vi "MoD Main-Optimize - HPLC - SUZUKI 04122017.vi"() -> ()   [LabVIEW 2015]
uses:
  <vilib>/ni845x/ni845x.llb/ni845xControl.ctl
  <vilib>/MakerHub/LINX/Public/Peripherals/Analog/Analog Read 1 Chan.vi
  <vilib>/MakerHub/LINX/Public/Peripherals/Analog/Analog Read N Chans.vi
  <vilib>/MakerHub/LINX/Public/Peripherals/Digital/Digital Write 1 Chan.vi
  <vilib>/MakerHub/LINX/Private/Local IO/LinxAnalogRead.vi
  <vilib>/MakerHub/LINX/Public/Utilities/Check Channel.vi
  <vilib>/MakerHub/LINX/Public/Peripherals/Digital/Digital Write N Chans.vi
  <vilib>/MakerHub/LINX/Private/Local IO/LinxDigitalWrite.vi
  <vilib>/addons/control/pid/pid.llb/PID Control Input Filter (DBL).vi
  <vilib>/MakerHub/LINX/Private/Utilties/Generate Error.vi
  <vilib>/addons/control/pid/autopid.llb/PID Online Autotuning (Relay Feedback).vi
  <vilib>/ni845x/ni845x.llb/NI-845x Close Device Reference.vi
  <vilib>/MakerHub/LINX/LMH-LINX.lvlib
  <vilib>/addons/control/pid/NI_PID_autopid.lvlib
  <vilib>/addons/control/pid/NI_PID_pid.lvlib
  <instrlib>/Harvard Apparatus PHD Ultra Series/Harvard Apparatus PHD Ultra Series.lvlib
panel:
  in  "Debug_run_button":bool
  out "Phase_Sensor_voltage":dbl
  out "P_tot":dbl
  out "pause for ms":bool=TRUE
  out "stop_xl_write":bool=TRUE
  out "Num_exp_till_pause":i32
  out "Syringe_pump?":bool=TRUE
  out "System Error":bool=TRUE
  out "error out":errorcluster
  out "Pump setpoint(ul/min) 6":dbl format="%#_13g"
  out "Pump setpoint(ul/min) 5":dbl format="%#_13g"
  out "Pump setpoint(ul/min) 4":dbl format="%#_13g"
  out "Pump setpoint(ul/min) 3":dbl format="%#_13g"
  out "Pump setpoint(ul/min) 2":dbl format="%#_13g"
  out "Pump setpoint(ul/min) 1":dbl format="%#_13g"
  out "Volume (ul) 5":dbl format="%#_13g"
  out "Volume (ul) 4":dbl format="%#_13g"
  out "Volume (ul) 3":dbl format="%#_13g"
  out "Volume (ul) 2":dbl format="%#_13g"
  out "Volume (ul) 1":dbl format="%#_13g"
  in  "tau 5":dbl format="%#_13g"
  out "tau 4":dbl format="%#_13g"
  out "tau 3":dbl format="%#_13g"
  out "tau 2":dbl format="%#_13g"
  out "tau 1":dbl format="%#_13g"
  out "Reactor Length":dbl format="%#_13g"
  out "Flowrate Sensor 2":dbl format="%#_13g"
  out "Flowrate Sensor 1":dbl format="%#_13g"
  out "Pressure 2":dbl format="%#_13g"
  out "Pressure 1":dbl format="%#_13g"
  out "Temperature Control 5":bool=TRUE
  out "Temperature Control 4":bool=TRUE
  out "Temperature Control 3":bool=TRUE
  out "Temperature Control 2":bool=TRUE
  out "Temperature Control 1":bool=TRUE
  out "Temperature SP 5":dbl format="%#_g'C"
  out "Temperature SP 4":dbl format="%#_g'C"
  out "Temperature SP 3":dbl format="%#_g'C"
  out "Temperature SP 2":dbl format="%#_g'C"
  out "Temperature SP 1":dbl format="%#_g'C"
  in  "Bay Temperature 5":dbl
  in  "SSR Duration 5":dbl
  in  "SSR Duration 4":dbl
  in  "SSR Duration 3":dbl
  in  "SSR Duration 2":dbl
  in  "SSR Duration 1":dbl
  in  "Total Product Amount":dbl=1.0 format="%#_gml"
  out "Setup Error":bool=TRUE
  out "Error Message":string
  out "ID CTR":i32
  in  "Tab Control 2":enum32{"Faults", "Devices"}(tab)=enum."Devices"
  out "Fault Cluster":T1
  in  "COMM Port:: Harvard Syringe Pump":refnum<visa-resource-name>="COM5"
  in  "Sample Valve COMM::Port":refnum<visa-resource-name>="COM6"
  in  "Arduino COMM Port":refnum<visa-resource-name>="COM3"
  in  "COMM Port :: Milligat Pumps":refnum<visa-resource-name>="COM10"
  in  "IR Sensor Device":T2="USB0::0x3923::0x7514::01B3FF21::RAW"
  in  "Tab Control":enum32{"Setup", "Parameters", "Monitoring"}(tab)
  in  "System decide help Button":bool
  in  "Reaction Scheme Confirm":bool
  in  "Synthesis Route Array":string[](array[string])=["3-Br-Pyridine _ Biphenyl", "K2CO3", "PhB(OH)2", "", "", ""]
  in  "Manual/Automated":bool
  in  "Save Button":bool
  in  "Open Button":bool
  in  "New rxn scheme button":bool
  in  "System decide help Button 2":bool
  out "Setup Confirm":bool=TRUE
  in  "BAY 1":u16(ring) items=["                 Bypass", "             Hot Reactor", "               Separator"]
  in  "BAY 5":u16(ring) items=["                     Bypass", "                Hot Reactor", "                 Separator"]
  in  "BAY 4":u16(ring) items=["                     Bypass", "                Hot Reactor", "                  Separator"]
  in  "BAY 3":u16(ring)=1 items=["                     Bypass", "                 Hot Reactor", "                  Separator"]
  in  "BAY 2":u16(ring) items=["                     Bypass", "                Hot Reactor", "                  Separator"]
  in  "System Parameters Help Button":bool
  in  "System Parameters Confirm Button":bool
  in  "Bay Parameters":T3={"Pump 1 Reagent Concentration"=0.8, "Pump 2 Reagent Concentration"=0.55, "Pump 3 Reagent Concentration"=0.4, "Pump 4 Reagent Concentration"=0.0, "Pump 5 Reagent Concentration"=0.0, "Bay 1 Parameters"={"Pump 1 Flowrate"=0.0, "optimize_temp"=FALSE, "optimize_tau"=TRUE, "Run at set flowrate"=FALSE, "Pump 2 Flowrate"=0.0, "Temperature Params"=[0.0, 40.0, 100.0], "pump params 1"=[0.0, 32.5, 325.0], "pump params 2"=[0.0, 32.5, 325.0]}, "Bay 2 Parameters"={"Pump 3 Flowrate"=0.0, "optimize_temp"=FALSE, "optimize_tau"=TRUE, "Run at set flowrate"=FALSE, "Temperature Params"=[0.0, 40.0, 100.0], "Resisdence time params"=[0.0, 65.0, 650.0], "pump_at_ratio"=FALSE, "pump_num_ratio"=0.0}, "Bay 3 Parameters"={"Pump 4 Flowrate"=0.0, "optimize_temp"=TRUE, "optimize_tau"=FALSE, "Run at set flowrate"=FALSE, "Temperature Params"=[0.0, 40.0, 100.0], "Resisdence time params"=[0.0, 0.0, 0.0], "pump_at_ratio"=FALSE, "pump_num_ratio"=0.0}, "Bay 4 Parameters"={"Pump 5 Flowrate"=40.0, "Run at set flowrate"=FALSE, "optimize_temp"=FALSE, "optimize_tau"=FALSE, "Resisdence time params"=[0.0, 36.0, 225.0], "Temperature Params"=[0.0, 40.0, 80.0], "pump_at_ratio"=FALSE, "pump_num_ratio"=0.0}, "Bay 5 Parameters"={"Pump 6 Flowrate"=0.0, "Run at set flowrate"=FALSE, "optimize_temp"=FALSE, "optimize_tau"=FALSE, "Resisdence time params"=[0.0, 0.0, 0.0], "Temperature Params"=[0.0, 0.0, 0.0], "pump_at_ratio"=FALSE, "pump_num_ratio"=0.2}, "Bay 1 Flow Rate Ratio \n(Pump 1: Pump 2)"=1.0, "tube_id(in)"=[enum.".02", enum.".03", enum.".03", enum.".03", enum.".03"], "xml_filename"="temp_xml", "Excel File Name"="C:\\Users\\HPLC\\Dropbox (MIT)\\MoD Files\\Data\\HWE Results\\SUZUKI Optimization HPLC - 04122017", "hplc File Name"="C:\\Chem32\\1\\Data\\MOD", "Matlab File"="C:\\Users\\HPLC\\Dropbox (MIT)\\MoD Files\\Data\\SUZUKI 04132017b", "Syringe for Pump 2?"=FALSE, "Num_conditons_per_wait"=1.0, "Continue from previous optimization?"=FALSE, "Pump 6 Reagent Concentration"=0.0, "Pause before analysis?"=FALSE, "Hplc Wait time(min)"=9.2} {"Hplc Wait time(min)" format="%#_13g"; "Pump 6 Reagent Concentration" format="%#_6gM"; "Bay 5 Parameters"."Temperature Params" format="%#_g'C"; "Bay 4 Parameters"."Temperature Params" format="%#_g'C"; "Bay 3 Parameters"."Temperature Params" format="%#_g'C"; "Bay 2 Parameters"."Temperature Params" format="%#_g'C"; "Bay 1 Parameters"."Temperature Params" format="%#_g'C"; "Pump 5 Reagent Concentration" format="%#_6gM"; "Pump 4 Reagent Concentration" format="%#_6gM"; "Pump 3 Reagent Concentration" format="%#_6gM"; "Pump 2 Reagent Concentration" format="%#_6gM"; "Pump 1 Reagent Concentration" format="%#_6gM"}
  out "System Confirm Not Clicked":string
  out "Setup Confirm 2":bool=TRUE
  out "Current Experiment":dbl
  in  "Total Number of Experiments":dbl=33.0
  out "Phase Sensor Chart":T4(graph)
  out "HPLC Analysis":bool
  out "Equlibrating Temperature":bool
  out "Flushing System":bool
  out "Calculate condition":bool
  out "System Flush Wait Time":u8(slide) scale=0.0..1149.042355163602
  out "Temperature 5":dbl format="%#_g'C"
  out "Temperature 4":dbl format="%#_g'C"
  out "Temperature 3":dbl format="%#_g'C"
  out "Temperature 2":dbl format="%#_g'C"
  out "Temperature 1":dbl format="%#_g'C"
  out "Flowrate Chart":T4(graph)
  out "Bay 5":u16(ring) items=["                     Bypass", "                   Reactor1", "               Separator"]
  out "Bay 4":u16(ring) items=["                     Bypass", "                   Reactor1", "               Separator"]
  out "Bay 3":u16(ring) items=["                     Bypass", "                   Reactor1", "               Separator"]
  out "Bay 2":u16(ring) items=["                     Bypass", "                   Reactor1", "               Separator"]
  out "Bay 1":u16(ring) items=["                     Bypass", "                   Reactor1", "               Separator"]
  out "Teperature Chart":T4(graph)
  out "Pump Setpoints Chart":T4(graph)
  out "Pressure Chart":T4(graph)
  out "Optimization_loop_index":i32
  out "curr_wait_time":dbl
  out "total_flush_time":dbl
  out "Temp SS? 5":bool=TRUE
  out "Temp SS? 4":bool=TRUE
  out "Temp SS? 3":bool=TRUE
  out "Temp SS? 2":bool=TRUE
  out "Temp SS? 1":bool=TRUE
  out "System Flushed?":bool
  out "stop_button clicked":bool
  out "Total System Resisdence Time(min)":dbl
  out "Stop":bool=TRUE
  in  "Run_Stop_cluster":T5
  # "Molecules on Demand"
  # "Synthesis Route"
  # "Reagent List"
  # "1"
  # "2"
  # "1"
  # "3"
  # "2"
  # "4"
  # "3"
  # "5"
  # "4"
  # "6"
  # "5"
  # "Product"
  # "6"
  # "Have system decide based on synthesis route"
  # "Manually enter bay configuration"
  # "System Schematic"
  # "Optimization Parameters"
  # "Bay"
  # "Tube ID (in)"
  # "1."
  # "2."
  # "3."
  # "4."
  # "5."
  # "Pause after"
  # "Experiments"
  # "Reporting"
  # "XML Output File Name"
  # "Excel Output File Name"
  # "HPLC File Path"
  # "MATLAB File Path"
  # "Temperature"
  # "Flowrate(ul/min)"
  # "Setpoint"
  # "Lower Bound"
  # "Upper Bound"
  # "Optimize?"
  # "-or-"
  # "Run at"
  # "times incoming flow"
  # "Temperature"
  # "Flowrate(ul/min)"
  # "Setpoint"
  # "Lower Bound"
  # "Upper Bound"
  # "Optimize?"
  # "-or-"
  # "Run at"
  # "times incoming flow"
  # "Temperature"
  # "Flowrate(ul/min)"
  # "Setpoint"
  # "Lower Bound"
  # "Upper Bound"
  # "Optimize?"
  # "-or-"
  # "Run at"
  # "times incoming flow"
  # "Temperature"
  # "Flowrate 3 (ul/min)"
  # "Setpoint"
  # "Lower Bound"
  # "Upper Bound"
  # "Optimize?"
  # "-or-"
  # "Run at"
  # "times incoming flow"
  # "Temperature"
  # "Flowrate 1(ul/min)"
  # "Flowrate 2(ul/min)"
  # "Setpoint"
  # "Lower Bound"
  # "Upper Bound"
  # "Optimize?"
  # "Temperature('C)"
  # "Pressure (psi)"
  # "Flowrate (ul/min)"
  # "Pump Flowrate Setpoints(ul/min)"
  # "Phase Sensor Value"
  # "Experimental Steps"
  # "Calculated new conditions"
  # "Flushed System"
  # "Analyzed HPLC"
  # "Equilibrated Temperature"
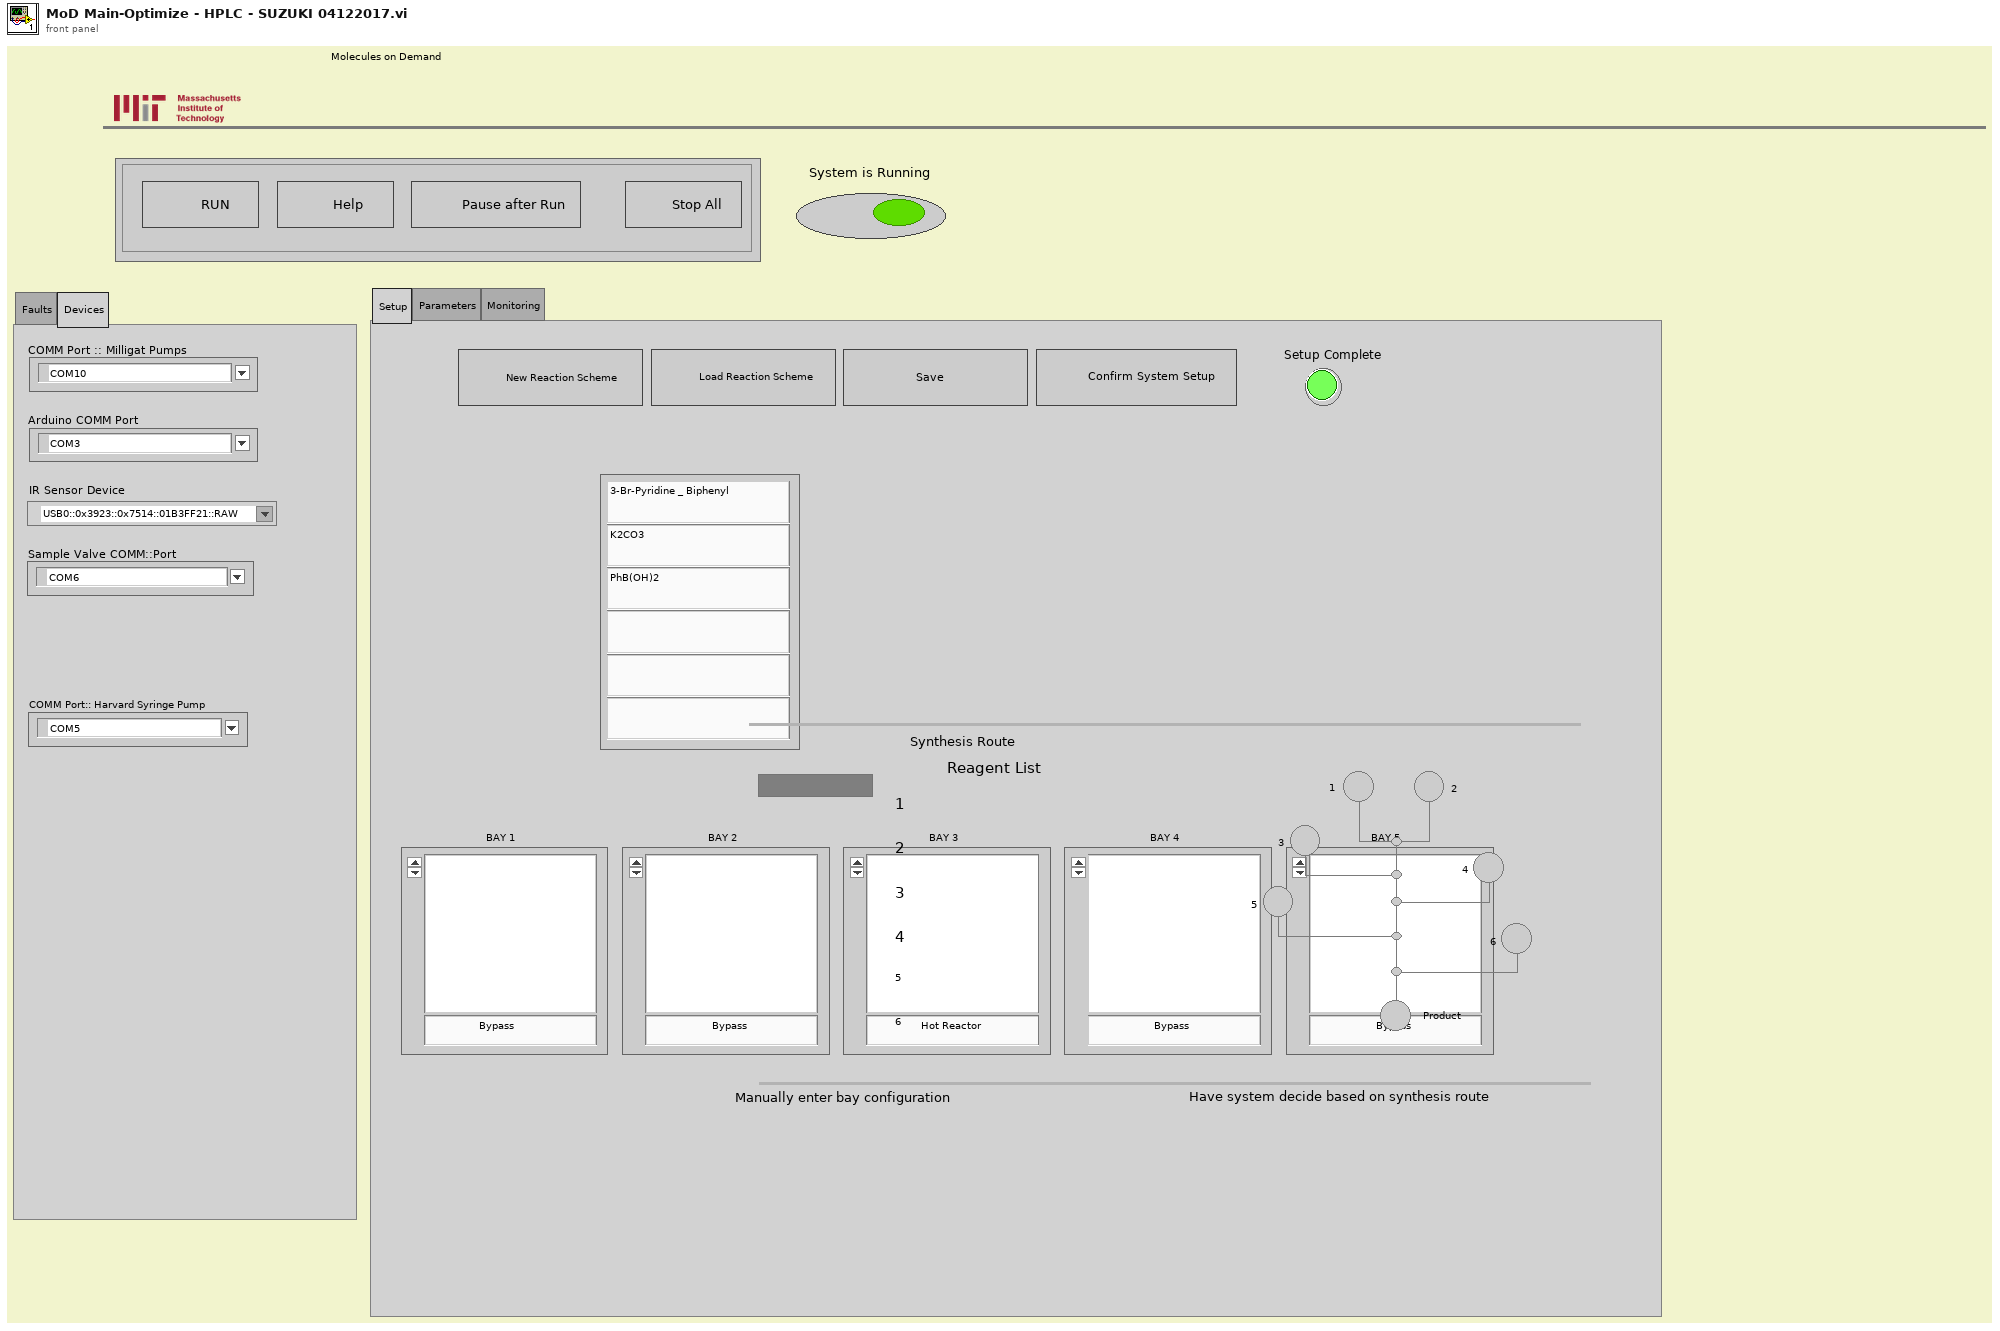
[diagram p1: front panel]
types:
  T1 = cluster{"Pump COMM Port":bool, "Pressure":bool, "Flow Rate":bool, "Temperature Sensor COMM Port":bool, "Arduino COMM Port":bool, "Chiller COMM Port":bool}
  T2 = typedef "ni845xControl.ctl" = refnum<k21>
  T3 = cluster{"Pump 1 Reagent Concentration":dbl, "Pump 2 Reagent Concentration":dbl, "Pump 3 Reagent Concentration":dbl, "Pump 4 Reagent Concentration":dbl, "Pump 5 Reagent Concentration":dbl, "Bay 1 Parameters":cluster{"Pump 1 Flowrate":dbl, "optimize_temp":bool, "optimize_tau":bool, "Run at set flowrate":bool, "Pump 2 Flowrate":dbl, "Temperature Params":dbl[], "pump params 1":dbl[], "pump params 2":dbl[]}, "Bay 2 Parameters":cluster{"Pump 3 Flowrate":dbl, "optimize_temp":bool, "optimize_tau":bool, "Run at set flowrate":bool, "Temperature Params":dbl[], "Resisdence time params":dbl[], "pump_at_ratio":bool, "pump_num_ratio":dbl}, "Bay 3 Parameters":cluster{"Pump 4 Flowrate":dbl, "optimize_temp":bool, "optimize_tau":bool, "Run at set flowrate":bool, "Temperature Params":dbl[], "Resisdence time params":dbl[], "pump_at_ratio":bool, "pump_num_ratio":dbl}, "Bay 4 Parameters":cluster{"Pump 5 Flowrate":dbl, "Run at set flowrate":bool, "optimize_temp":bool, "optimize_tau":bool, "Resisdence time params":dbl[], "Temperature Params":dbl[], "pump_at_ratio":bool, "pump_num_ratio":dbl}, "Bay 5 Parameters":cluster{"Pump 6 Flowrate":dbl, "Run at set flowrate":bool, "optimize_temp":bool, "optimize_tau":bool, "Resisdence time params":dbl[], "Temperature Params":dbl[], "pump_at_ratio":bool, "pump_num_ratio":dbl}, "Bay 1 Flow Rate Ratio \n(Pump 1: Pump 2)":dbl, "tube_id(in)":enum16{".01", ".02", ".03", ".04"}[], "xml_filename":string, "Excel File Name":string, "hplc File Name":string, "Matlab File":string, "Syringe for Pump 2?":bool, "Num_conditons_per_wait":dbl, "Continue from previous optimization?":bool, "Pump 6 Reagent Concentration":dbl, "Pause before analysis?":bool, "Hplc Wait time(min)":dbl}
  T4 = cluster{"[0]":dbl, "[1]":dbl, "[2]":dbl, "[3]":dbl, "[4]":dbl, "[5]":dbl, "[6]":dbl, "[7]":dbl, "[8]":dbl}
  T5 = cluster{"Stop":bool, "Help Button":bool, "Run":bool, "Stop Run Button":bool}
  T6 = cluster{"Proportional gain Kc":dbl, "Integral time Ti (sec)":dbl, "Derivative time Ti (sec)":dbl}
  T7 = cluster{"type of controller":enum16{"P", "PI", "PID"}, "relay cycles":i32, "relay amplitude":dbl, "control specifications":enum16{"Fast", "Normal", "Slow"}, "PV noise level":dbl}
  T8 = typedef "LMH-LINX.lvlib/LINX Ref.ctl" = cluster{"IO":T9, "Interface":T10, "LINX Device Config":T11}
  T9 = typedef "LMH-LINX.lvlib/Platform.ctl" = enum16{"Remote", "Local"}
  T10 = typedef "LMH-LINX.lvlib/Interface.ctl" = enum16{"Serial", "TCP"}
  T11 = typedef "LMH-LINX.lvlib/Device.lvlib/LINX Device Config.ctl" = cluster{"Interface":T10, "COM Port":refnum<visa-resource-name>, "TCP Configuration":T12, "Device Family":u8, "Device ID":u8, "Device Name":string, "TCP Ref":refnum<k5>, "Channels":T13}
  T12 = typedef "LMH-LINX.lvlib/Device.lvlib/TCP Config.ctl" = cluster{"IP Address":string, "Port":u16}
  T13 = typedef "LMH-LINX.lvlib/Channels.ctl" = cluster{"DI":u8[], "DO":u8[], "AI":u8[], "AO":u8[], "PWM":u8[], "QE":u8[], "UART":u8[], "I2C 2":u8[], "SPI":u8[], "CAN":u8[], "Servo":u8[], "AI Ref (V)":dbl, "AI Resolution (Bits)":u8, "AO Ref (V)":dbl, "AO Resolution (Bits)":u8}
  T14 = cluster{"proportional gain (Kc)":dbl, "integral time (Ti, min)":dbl, "derivative time (Td, min)":dbl}
  T15 = enum16{"Left Button", "Center Button", "Right Button", "Window Close"}
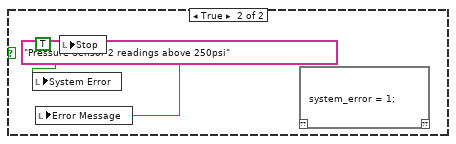
[diagram p2: hidden frame]
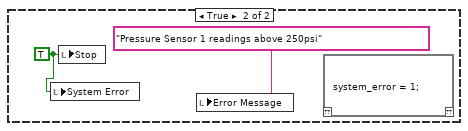
[diagram p3: hidden frame]
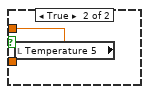
[diagram p4: hidden frame]
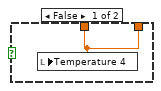
[diagram p5: hidden frame]
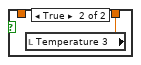
[diagram p6: hidden frame]
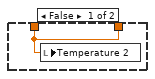
[diagram p7: hidden frame]
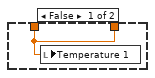
[diagram p8: hidden frame]
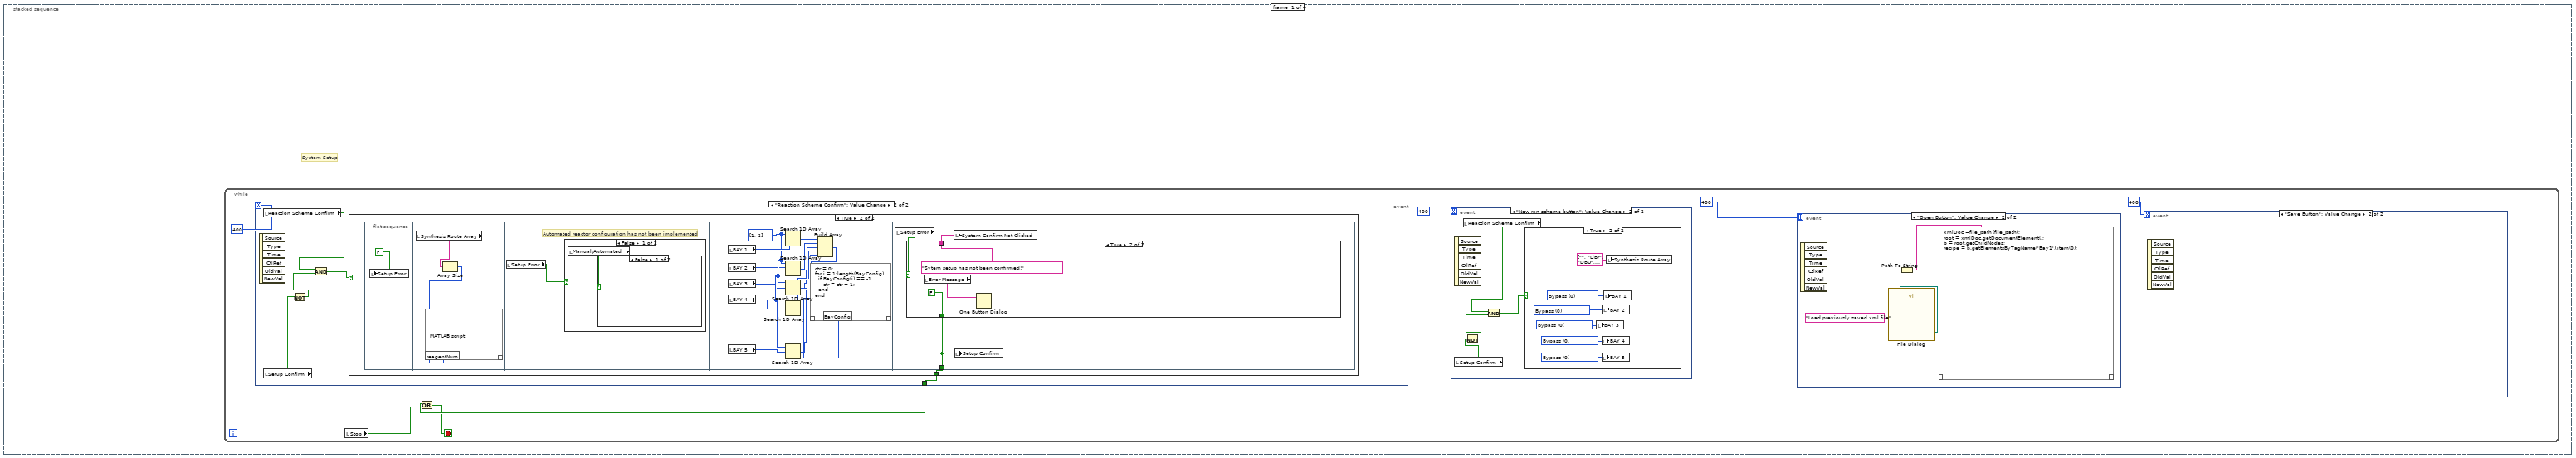
[diagram p9: hidden frame]
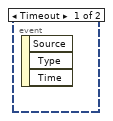
[diagram p10: hidden frame]
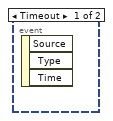
[diagram p11: hidden frame]
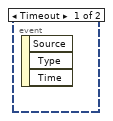
[diagram p12: hidden frame]
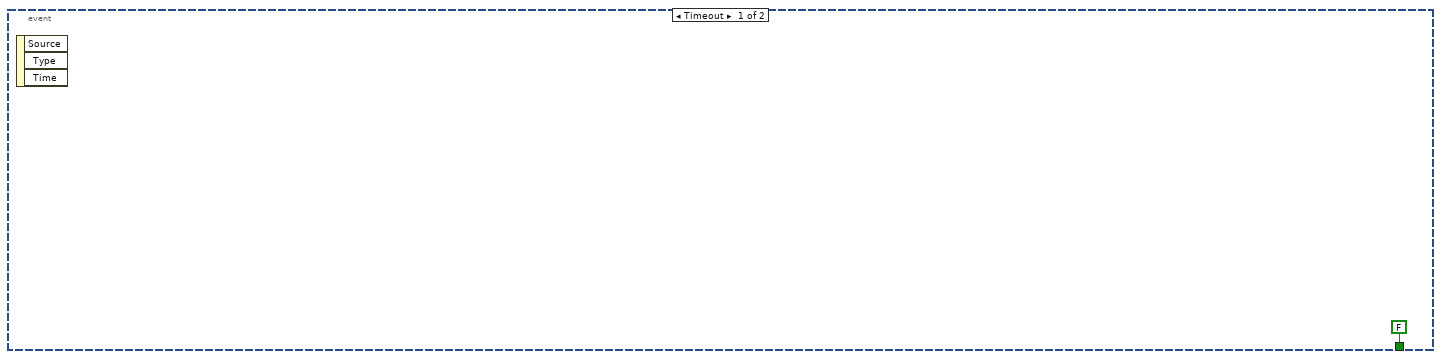
[diagram p14: hidden frame]
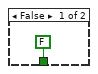
[diagram p15: hidden frame]
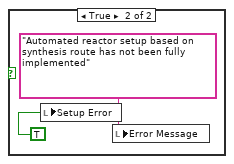
[diagram p16: hidden frame]
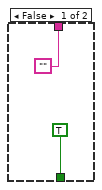
[diagram p18: hidden frame]
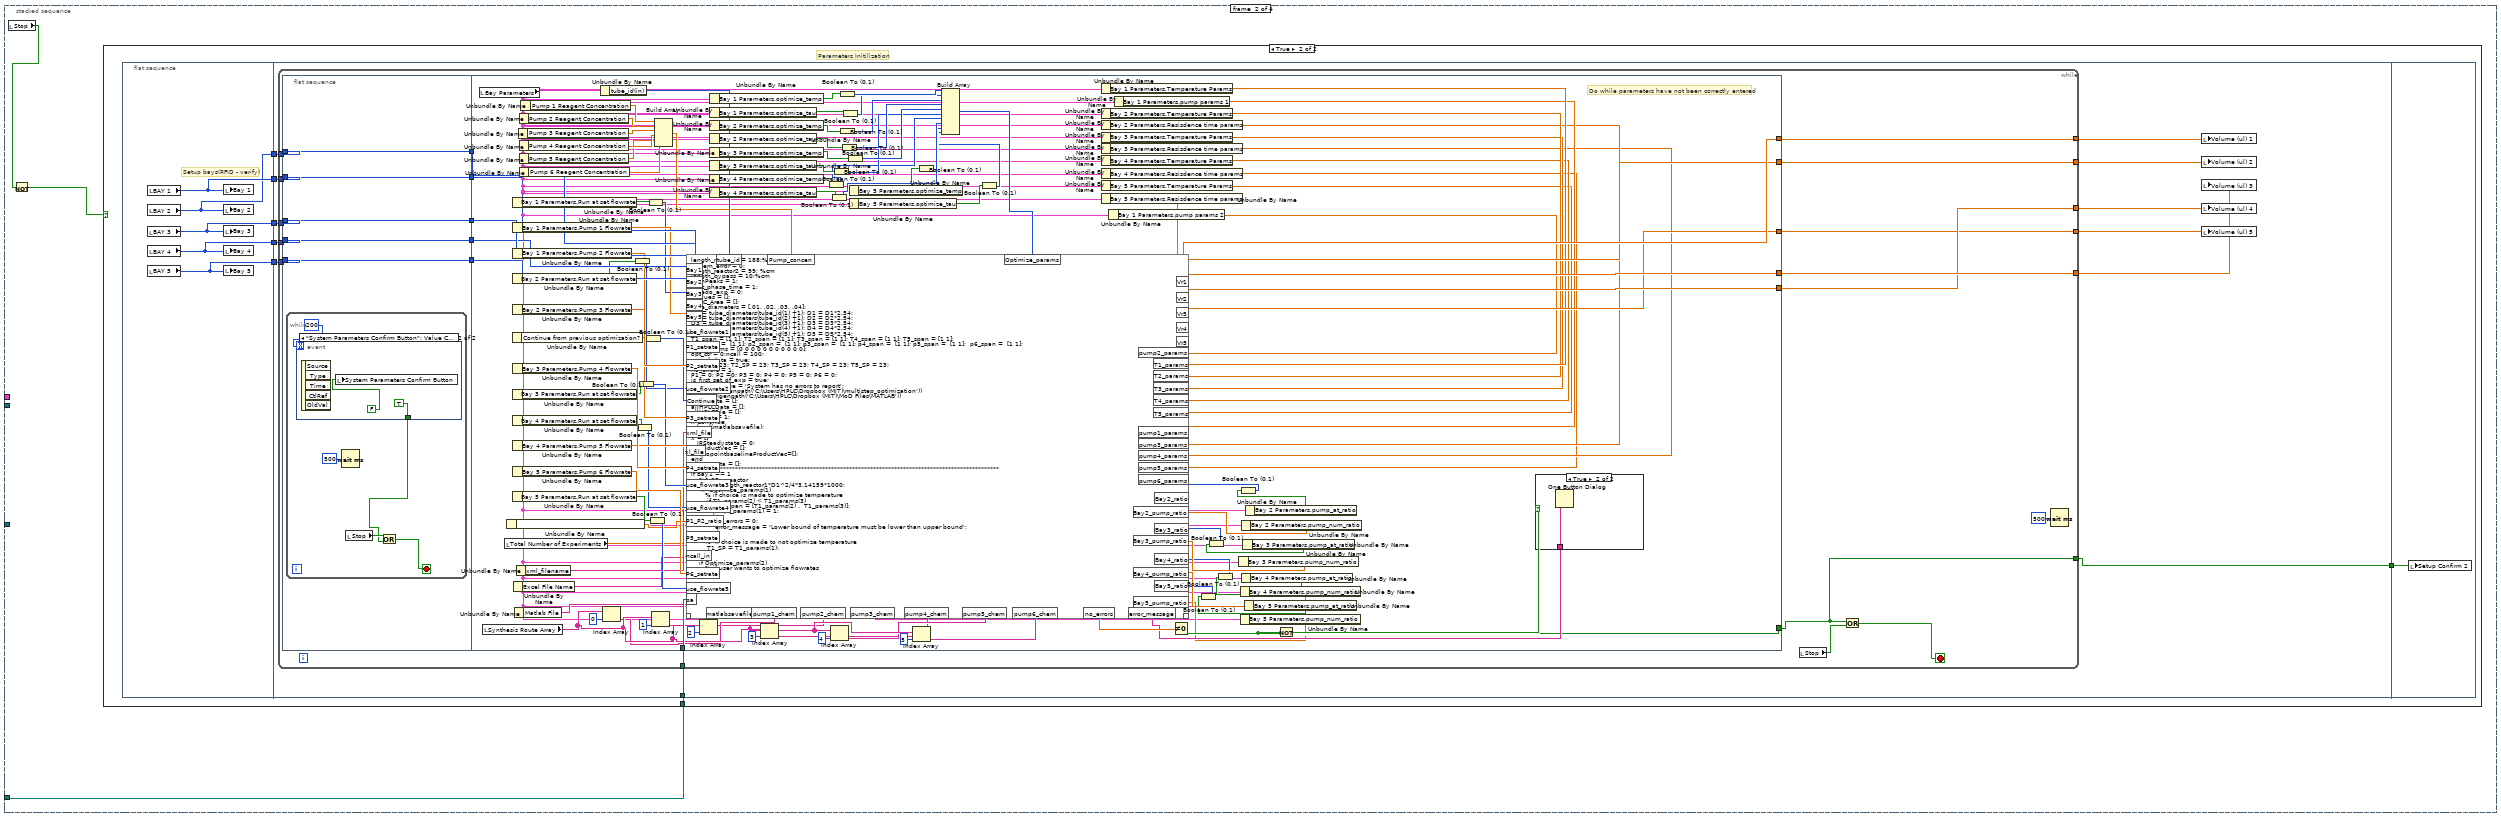
[diagram p19: hidden frame]
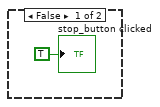
[diagram p20: hidden frame]
diagram:
  # "Assume User always uses the first bay first"
  n1 = flat-sequence {
    tunnel: ["COMM Port :: Milligat Pumps"] -> w10
    tunnel: ["Arduino COMM Port"] -> w9
    tunnel: [w12] -> w2
    tunnel: ["Bay Parameters"] -> w1
    tunnel: [w51] -> w11
    tunnel: w10 -> [w51]
    tunnel: w9 -> [w50]
    tunnel: [w44] -> w8
    tunnel: [w44] -> w7
    tunnel: [w32] -> w4
    tunnel: [w30] -> w3
    tunnel: w2 -> [w30]
    tunnel: w1 -> [w28]
    tunnel: w11 -> [w59]
    tunnel: w8 -> [w58]
    tunnel: w7 -> [w52]
    tunnel: [w57] -> w6
    tunnel: w4 -> [w56]
    tunnel: w3 -> [w53]
    tunnel: w6 -> [w1229]
    tunnel: [w1229] -> w5
    tunnel: w5 -> [w1236]
    frame #0 {
      w16 = FALSE ("Equlibrating Temperature")
      n2 = script code="TempArr1=[23 23 23 23 23 23 23 23 23 23]';\nTempArr2=[23 23 23 23 23 23 23 23 23 23]';\nTempArr3=[23 23 23 23 23 23 23 23 23 23]';\nTempArr4=[23 23 23 23 23 23 23 23 23 23]';\nTempArr5=[23 23 23 23 23 23 23 23 23 23]';\ntemp_error1 =0;\ntemp_error2 =0;\ntemp_error3 =0;\ntemp_error4 =0;\ntemp_error5 =0;\ntemp_check1 = 0;\ntemp_check2 = 0;\ntemp_check3 = 0;\ntemp_check4 = 0;\ntemp_check5 = 0;\nT1=23;\nT2=23;\nT3=23;\nT4=23;\nT5=23;"() -> ()  [unwired: 1 in, 1 out]
      n3 = call <vilib>:"Initialize.vi"("VISA resource name"="COMM Port:: Harvard Syringe Pump") -> ("VISA resource name out"=w12:refnum<visa-resource-name>)  [unwired: 9 in, 1 out]
      "Stop" <- FALSE ("Stop")
      "ID CTR" <- 0
      "Setup Confirm" <- FALSE ("Setup Confirm")
      "Setup Error" <- FALSE ("Setup Error")
      "Reactor Length" <- 10.5
      "System Error" <- FALSE ("System Error")
      "Num_exp_till_pause" <- 0 ("Num_exp_till_pause")
      "Equlibrating Temperature" <- w16
      "Calculate condition" <- w16
      "Flushing System" <- w16
      "HPLC Analysis" <- w16
      "Setup Confirm 2" <- FALSE ("Setup Confirm 2")
      "stop_xl_write" <- FALSE ("stop_xl_write")
    }
    frame #1 {
      w43 = 23
      (unwired) path "C:/Users/User1/Documents/Lab/MoD/Images"
      n4 = local write "Debug_run_button"(TRUE) -> ()
      n5 = local read "BAY 2"() -> (w48:u16)
      n6 = local read "BAY 3"() -> (w47:u16)
      n7 = local read "BAY 4"() -> (w46:u16)
      n8 = local read "BAY 5"() -> (w45:u16)
      n9 = local read "BAY 1"() -> (w49:u16)
      n10 = local write "Bay 1"(w49) -> ()
      n11 = local write "Bay 2"(w48) -> ()
      n12 = local write "Bay 3"(w47) -> ()
      n13 = local write "Bay 4"(w46) -> ()
      n14 = local write "BAY 5"(w45) -> ()
      n15 = call <vilib>:"Initialize.vi"("Serial Port"=w50) -> ("LINX Resource"=w44:T8)  [unwired: 8 in, 2 out]
      n16 = Unbundle By Name(w28) -> ("Syringe for Pump 2?"=→"Syringe_pump?":bool)
      n17 = local write "Temperature 1"(w43) -> ()
      n18 = local write "Temperature 2"(w43) -> ()
      n19 = local write "Temperature 3"(w43) -> ()
      n20 = local write "Temperature 4"(w43) -> ()
      n21 = local write "Temperature 5"(w43) -> ()
      n22 = local write "Temperature SP 1"(w43) -> ()
      n23 = local write "Temperature SP 2"(w43) -> ()
      n24 = local write "Temperature SP 3"(w43) -> ()
      n25 = local write "Temperature SP 4"(w43) -> ()
      n26 = local write "Temperature SP 5"(w43) -> ()
      n27 = Unbundle By Name(w28) -> ("Pause before analysis?"=→"pause for ms":bool)
      n28 = Current VI's Path() -> (path=w36:path)
      n29 = Strip Path(path=w36) -> (stripped path=w34:path)  [unwired: 1 out]
      n30 = Strip Path(path=w34) -> (stripped path=w33:path)  [unwired: 1 out]
      n31 = Build Path(base path=w33, name or relative path="MATLAB") -> (appended path=w32:path)
      "Pump setpoint(ul/min) 1" <- 0.0 ("Pump setpoint(ul/min) 1")
      "Pump setpoint(ul/min) 2" <- 0.0 ("Pump setpoint(ul/min) 2")
      "Pump setpoint(ul/min) 3" <- 0.0 ("Pump setpoint(ul/min) 3")
      "Pump setpoint(ul/min) 4" <- 0.0 ("Pump setpoint(ul/min) 4")
      "Pump setpoint(ul/min) 5" <- 0.0 ("Pump setpoint(ul/min) 5")
      "Pump setpoint(ul/min) 6" <- 0.0 ("Pump setpoint(ul/min) 6")
    }
    frame #2 {
      # "Main Help Dialog Popup"
      n32 = while {
        stop <- w1224 stop-if-true
        n33 = event shown="[1] \"Run_Stop_cluster.Help Button\": Value Change" {
          selector: _ -> [_ _ _ _ _ _]
          dyn-events: _ -> [_ _ _ _ _ _]
          timeout: 100 -> [_ _ _ _ _ _]
          event Timeout {
            n34 = event-data() -> ()  [unwired: 1 in, 3 out]
          }
          event "Run_Stop_cluster.Help Button": Value Change {
            n35 = local read "Run_Stop_cluster"() -> (w1227:T5)
            n36 = event-data() -> ()  [unwired: 1 in, 4 out]
            n37 = Unbundle By Name(w1227) -> ("Help Button"=w1226:bool)
            n38 = case shown="True" w1226 {
              frame False {
              }
              frame True {
                n39 = call "help.vi"() -> ()  [unwired: 11 in]
              }
            }
          }
          event "System decide help Button": Value Change {
            n40 = event-data() -> ()  [unwired: 1 in, 5 out]
            n41 = call "help_synthesis_man-auto_instructions.vi"() -> ()  [unwired: 12 in]
          }
          event "System Parameters Help Button": Value Change {
            n42 = event-data() -> ()  [unwired: 1 in, 5 out]
            n43 = call "help_parameters_setup.vi"() -> ()  [unwired: 12 in]
          }
          event "System decide help Button 2": Value Change {
            n44 = event-data() -> ()  [unwired: 1 in, 5 out]
            n45 = call "help_synthesis_route_instructions.vi"() -> ()  [unwired: 12 in]
          }
          event "Run_Stop_cluster.Stop": Value Change {
            n46 = event-data() -> ()  [unwired: 1 in, 5 out]
            n47 = local write "Stop"(TRUE) -> ()
          }
        }
        n48 = local read "Stop"() -> (w1224:bool)
      }
      n49 = stacked-sequence {
        tunnel: w59 -> [_ _ _ _]
        tunnel: w58 -> [_ _ _ w424]
        tunnel: [_ _ _ w424] -> w57
        tunnel: w56 -> [_ w258 _ _]
        tunnel: w53 -> [_ _ _ w425]
        frame #0 {
          # "System Setup"
          n50 = while {
            stop <- w204 stop-if-true
            n51 = event shown="[1] \"Reaction Scheme Confirm\": Value Change" {
              selector: _ -> [_ _]
              dyn-events: _ -> [_ _]
              timeout: 400 -> [_ _]
              tunnel: [FALSE w222] -> w206
              event Timeout {
                n52 = event-data() -> ()  [unwired: 1 in, 3 out]
              }
              event "Reaction Scheme Confirm": Value Change {
                n53 = event-data() -> ()  [unwired: 1 in, 6 out]
                n54 = local read "Reaction Scheme Confirm"() -> (w226:bool)
                n55 = local read "Setup Confirm"() -> (w224:bool)
                n56 = Not(x=w224) -> (.not. x?=w223:bool)
                n57 = And(x=w226, y=w223) -> (x .and. y?=w225:bool)
                n58 = case shown="True" w225 {
                  tunnel: [FALSE w228] -> w222
                  frame False {
                  }
                  frame True {
                    n59 = flat-sequence {
                      tunnel: [w248] -> w228
                      frame #0 {
                        n60 = local write "Setup Error"(FALSE) -> ()
                      }
                      frame #1 {
                        n61 = local read "Synthesis Route Array"() -> (w231:string[])
                        n62 = Array Size(array=w231) -> (size(s)=w230:i32)
                        n63 = script code="MATLAB script"("reagentNum"=w230) -> ()  [unwired: 1 in, 1 out]
                      }
                      frame #2 {
                        # "Automated reactor configuration has not been implemented"
                        n64 = local read "Setup Error"() -> (w232:bool)
                        n65 = case shown="False" w232 {
                          frame False {
                            n66 = local read "Manual/Automated"() -> (w233:bool)
                            n67 = case shown="False" w233 {
                              frame False {
                              }
                              frame True {
                                n68 = local write "Setup Error"(TRUE ("Setup Error")) -> ()
                                n69 = local write "Error Message"("Automated reactor setup based on synthesis route has not been fully implemented") -> ()
                              }
                            }
                          }
                          frame True {
                          }
                        }
                      }
                      frame #3 {
                        w246 = i32[] [1, 2]
                        n70 = local read "BAY 1"() -> (w247:u16)
                        n71 = local read "BAY 2"() -> (w245:u16)
                        n72 = local read "BAY 3"() -> (w244:u16)
                        n73 = local read "BAY 4"() -> (w243:u16)
                        n74 = local read "BAY 5"() -> (w242:u16)
                        n75 = Search 1D Array(1D array=w246, element=w247) -> (index of element=w241:i32)  [unwired: 1 in]
                        n76 = Search 1D Array(1D array=w246, element=w245) -> (index of element=w240:i32)  [unwired: 1 in]
                        n77 = Search 1D Array(1D array=w246, element=w244) -> (index of element=w239:i32)  [unwired: 1 in]
                        n78 = Search 1D Array(1D array=w246, element=w243) -> (index of element=w238:i32)  [unwired: 1 in]
                        n79 = Search 1D Array(1D array=w246, element=w242) -> (index of element=w237:i32)  [unwired: 1 in]
                        n80 = Build Array(w241, w240, w239, w238, w237) -> (w236:i32[])
                        n81 = script code="ctr = 0;\nfor i = 1:length(BayConfig)\n  if BayConfig(i) == -1\n     ctr = ctr + 1;\n  end\nend"("BayConfig"=w236) -> ()  [unwired: 1 in, 1 out]
                      }
                      frame #4 {
                        n82 = local read "Setup Error"() -> (w250:bool)
                        n83 = case shown="True" w250 {
                          tunnel: [TRUE FALSE] -> w248
                          tunnel: ["" "Sytem setup has not been confirmed!"] -> w249
                          frame False {
                          }
                          frame True {
                            n84 = local read "Error Message"() -> (w255:string)
                            n85 = One Button Dialog(message=w255) -> ()  [unwired: 1 in, 1 out]
                          }
                        }
                        n86 = local write "System Confirm Not Clicked"(w249) -> ()
                        n87 = local write "Setup Confirm"(w248) -> ()
                      }
                    }
                  }
                }
              }
            }
            n88 = local read "Stop"() -> (w205:bool)
            n89 = Or(x=w206, y=w205) -> (x .or. y?=w204:bool)
            n90 = event shown="[1] \"New rxn scheme button\": Value Change" {
              selector: _ -> [_ _]
              dyn-events: _ -> [_ _]
              timeout: 400 -> [_ _]
              event Timeout {
                n91 = event-data() -> ()  [unwired: 1 in, 3 out]
              }
              event "New rxn scheme button": Value Change {
                n92 = event-data() -> ()  [unwired: 1 in, 6 out]
                n93 = local read "Setup Confirm"() -> (w211:bool)
                n94 = local read "Reaction Scheme Confirm"() -> (w212:bool)
                n95 = Not(x=w211) -> (.not. x?=w214:bool)
                n96 = And(x=w212, y=w214) -> (x .and. y?=w213:bool)
                n97 = case shown="True" w213 {
                  frame False {
                  }
                  frame True {
                    w215 = u16 0 items=["                     Bypass", "                Hot Reactor", "                 Separator"] ("BAY 5")
                    w216 = u16 0 items=["                     Bypass", "                Hot Reactor", "                  Separator"] ("BAY 4")
                    w217 = u16 0 items=["                     Bypass", "                 Hot Reactor", "                  Separator"] ("BAY 3")
                    w218 = u16 0 items=["                     Bypass", "                Hot Reactor", "                  Separator"] ("BAY 2")
                    w219 = u16 0 items=["                 Bypass", "             Hot Reactor", "               Separator"] ("BAY 1")
                    n98 = local write "BAY 3"(w217) -> ()
                    n99 = local write "BAY 4"(w216) -> ()
                    n100 = local write "BAY 5"(w215) -> ()
                    n101 = local write "BAY 2"(w218) -> ()
                    n102 = local write "BAY 1"(w219) -> ()
                    n103 = local write "Synthesis Route Array"(string[] ["", "LiBr", "DBU", "Aldehyde", "Water", "Toluene"] ("Synthesis Route Array")) -> ()
                  }
                }
              }
            }
            n104 = event shown="[1] \"Open Button\": Value Change" {
              selector: _ -> [_ _]
              dyn-events: _ -> [_ _]
              timeout: 400 -> [_ _]
              event Timeout {
                n105 = event-data() -> ()  [unwired: 1 in, 3 out]
              }
              event "Open Button": Value Change {
                n106 = event-data() -> ()  [unwired: 1 in, 6 out]
                n107 = call "File Dialog"("prompt"="Load previously saved xml file") -> ("selected path"=w209:path)  [unwired: 11 in, 3 out]
                n108 = Path To String(path=w209) -> (string=w208:string)
                n109 = script code="xmlDoc = xmlread(file_path);\nroot = xmlDoc.getDocumentElement();\nb = root.getChildNodes;\nrecipe = b.getElementsByTagName('Bay1').item(0);"("file_path"=w208) -> ()  [unwired: 1 in, 1 out]
              }
            }
            n110 = event shown="[1] \"Save Button\": Value Change" {
              selector: _ -> [_ _]
              dyn-events: _ -> [_ _]
              timeout: 400 -> [_ _]
              event Timeout {
                n111 = event-data() -> ()  [unwired: 1 in, 3 out]
              }
              event "Save Button": Value Change {
                n112 = event-data() -> ()  [unwired: 1 in, 6 out]
              }
            }
          }
        }
        frame #1 {
          n113 = local read "Stop"() -> (w257:bool)
          n114 = Not(x=w257) -> (.not. x?=w256:bool)
          n115 = case shown="True" w256 {
            tunnel: w258 -> [_ w261]
            frame False {
              "stop_button clicked" <- TRUE ("stop_button clicked")
            }
            frame True {
              # "Parameters Initilization"
              n116 = flat-sequence {
                tunnel: [w271] -> w266
                tunnel: [w270] -> w265
                tunnel: [w269] -> w264
                tunnel: [w268] -> w263
                tunnel: [w267] -> w262
                tunnel: w266 -> [w283]
                tunnel: w265 -> [w282]
                tunnel: w264 -> [w281]
                tunnel: w263 -> [w280]
                tunnel: w262 -> [w279]
                tunnel: w261 -> [w273]
                tunnel: [w272] -> w260
                tunnel: w260 -> [w422]
                frame #0 {
                  # "Setup bays(RFID - verify)"
                  n117 = local read "BAY 1"() -> (w271:u16)
                  n118 = local read "BAY 2"() -> (w270:u16)
                  n119 = local read "BAY 3"() -> (w269:u16)
                  n120 = local read "BAY 4"() -> (w268:u16)
                  n121 = local read "BAY 5"() -> (w267:u16)
                  n122 = local write "Bay 1"(w271) -> ()
                  n123 = local write "Bay 2"(w270) -> ()
                  n124 = local write "Bay 3"(w269) -> ()
                  n125 = local write "Bay 4"(w268) -> ()
                  n126 = local write "Bay 5"(w267) -> ()
                }
                frame #1 {
                  n127 = while {
                    tunnel: w283 -> [w303]
                    tunnel: w282 -> [w302]
                    tunnel: w281 -> [w301]
                    tunnel: w280 -> [w300]
                    tunnel: w279 -> [w299]
                    tunnel: [w298] -> w278
                    tunnel: [w297] -> w277
                    tunnel: [w296] -> w276
                    tunnel: [w295] -> w275
                    tunnel: [w294] -> w274
                    tunnel: w273 -> [w285]
                    tunnel: [w284] -> w272
                    stop <- w293 stop-if-true
                    n128 = flat-sequence {
                      tunnel: w299 -> [w304]
                      tunnel: w300 -> [w305]
                      tunnel: w301 -> [w306]
                      tunnel: w302 -> [w307]
                      tunnel: w303 -> [w308]
                      tunnel: [w308] -> w290
                      tunnel: [w307] -> w289
                      tunnel: [w306] -> w288
                      tunnel: [w305] -> w287
                      tunnel: [w304] -> w286
                      tunnel: [w408] -> w298
                      tunnel: [w407] -> w297
                      tunnel: [w406] -> w296
                      tunnel: [w405] -> w295
                      tunnel: [w404] -> w294
                      tunnel: [w360] -> w284
                      tunnel: w290 -> [w420]
                      tunnel: w289 -> [w419]
                      tunnel: w288 -> [w418]
                      tunnel: w287 -> [w417]
                      tunnel: w286 -> [w416]
                      tunnel: w285 -> [w356]
                      frame #0 {
                        n129 = while {
                          stop <- w312 stop-if-true
                          n130 = event shown="[1] \"System Parameters Confirm Button\": Value Change" {
                            selector: _ -> [_ _]
                            dyn-events: _ -> [_ _]
                            timeout: u32 200 ("milliseconds to wait") -> [_ _]
                            tunnel: [FALSE TRUE] -> w310
                            event Timeout {
                              n131 = event-data() -> ()  [unwired: 1 in, 3 out]
                            }
                            event "System Parameters Confirm Button": Value Change {
                              n132 = event-data() -> ()  [unwired: 1 in, 5 out]
                              n133 = local write "System Parameters Confirm Button"(FALSE) -> ()
                            }
                          }
                          n134 = Wait (ms)(milliseconds to wait=u32 500) -> ()  [unwired: 1 out]
                          n135 = local read "Stop"() -> (w313:bool)
                          n136 = Or(x=w313, y=w310) -> (x .or. y?=w312:bool)
                        }
                      }
                      frame #1 {
                        # "Do while parameters have not been correctly entered"
                        n137 = local read "Bay Parameters"() -> (w318:T3)
                        n138 = local read "Synthesis Route Array"() -> (w333:string[])
                        n139 = local read "Total Number of Experiments"() -> (w319:dbl)
                        n140 = Unbundle By Name(w318) -> ("Bay 1 Flow Rate Ratio \n(Pump 1: Pump 2)"=w359:dbl)
                        n141 = Unbundle By Name(w318) -> ("Continue from previous optimization?"=w355:bool)
                        n142 = Unbundle By Name(w318) -> ("Bay 1 Parameters.Run at set flowrate"=w403:bool)
                        n143 = Unbundle By Name(w318) -> ("Bay 1 Parameters.Pump 1 Flowrate"=w414:dbl)
                        n144 = Unbundle By Name(w318) -> ("Bay 1 Parameters.Pump 2 Flowrate"=w413:dbl)
                        n145 = Unbundle By Name(w318) -> ("Bay 2 Parameters.Run at set flowrate"=w401:bool)
                        n146 = Unbundle By Name(w318) -> ("Bay 2 Parameters.Pump 3 Flowrate"=w412:dbl)
                        n147 = Unbundle By Name(w318) -> ("Bay 3 Parameters.Pump 4 Flowrate"=w411:dbl)
                        n148 = Unbundle By Name(w318) -> ("Bay 3 Parameters.Run at set flowrate"=w400:bool)
                        n149 = Unbundle By Name(w318) -> ("Bay 4 Parameters.Run at set flowrate"=w397:bool)
                        n150 = Unbundle By Name(w318) -> ("Bay 4 Parameters.Pump 5 Flowrate"=w410:dbl)
                        n151 = Unbundle By Name(w318) -> ("Bay 5 Parameters.Pump 6 Flowrate"=w409:dbl)
                        n152 = Unbundle By Name(w318) -> ("Bay 5 Parameters.Run at set flowrate"=w396:bool)
                        n153 = Unbundle By Name(w318) -> ("Excel File Name"=w357:string)
                        n154 = Unbundle By Name(w318) -> ("Matlab File"=w353:string)
                        n155 = Unbundle By Name(w318) -> ("xml_filename"=w358:string)
                        n156 = Unbundle By Name(w318) -> ("Pump 3 Reagent Concentration"=w324:dbl)
                        n157 = Unbundle By Name(w318) -> ("Pump 2 Reagent Concentration"=w325:dbl)
                        n158 = Unbundle By Name(w318) -> ("Pump 4 Reagent Concentration"=w323:dbl)
                        n159 = Unbundle By Name(w318) -> ("Pump 5 Reagent Concentration"=w322:dbl)
                        n160 = Unbundle By Name(w318) -> ("Pump 6 Reagent Concentration"=w321:dbl)
                        n161 = Unbundle By Name(w318) -> ("Pump 1 Reagent Concentration"=w326:dbl)
                        n162 = Unbundle By Name(w318) -> ("tube_id(in)"=w415:enum16{".01", ".02", ".03", ".04"}[])
                        n163 = Index Array(array=w333, index=0) -> (element=w332:string)
                        n164 = Boolean To (0,1)(Boolean=w401) -> (0, 1=w352:i16)
                        n165 = Boolean To (0,1)(Boolean=w397) -> (0, 1=w398:i16)
                        n166 = Boolean To (0,1)(Boolean=w400) -> (0, 1=w399:i16)
                        n167 = Boolean To (0,1)(Boolean=w355) -> (0, 1=w354:i16)
                        n168 = Boolean To (0,1)(Boolean=w403) -> (0, 1=w402:i16)
                        n169 = Boolean To (0,1)(Boolean=w396) -> (0, 1=w395:i16)
                        n170 = Index Array(array=w333, index=1) -> (element=w327:string)
                        n171 = Build Array(w326, w325, w324, w323, w322, w321) -> (w320:dbl[])
                        n172 = Index Array(array=w333, index=2) -> (element=w328:string)
                        n173 = Unbundle By Name(w318) -> ("Bay 1 Parameters.optimize_temp"=w394:bool)
                        n174 = Unbundle By Name(w318) -> ("Bay 1 Parameters.optimize_tau"=w392:bool)
                        n175 = Unbundle By Name(w318) -> ("Bay 2 Parameters.optimize_temp"=w390:bool)
                        n176 = Unbundle By Name(w318) -> ("Bay 2 Parameters.optimize_tau"=w388:bool)
                        n177 = Unbundle By Name(w318) -> ("Bay 3 Parameters.optimize_temp"=w386:bool)
                        n178 = Unbundle By Name(w318) -> ("Bay 3 Parameters.optimize_tau"=w384:bool)
                        n179 = Unbundle By Name(w318) -> ("Bay 4 Parameters.optimize_temp"=w382:bool)
                        n180 = Unbundle By Name(w318) -> ("Bay 4 Parameters.optimize_tau"=w380:bool)
                        n181 = Index Array(array=w333, index=3) -> (element=w329:string)
                        n182 = Boolean To (0,1)(Boolean=w382) -> (0, 1=w381:i16)
                        n183 = Boolean To (0,1)(Boolean=w380) -> (0, 1=w379:i16)
                        n184 = Index Array(array=w333, index=4) -> (element=w330:string)
                        n185 = Boolean To (0,1)(Boolean=w384) -> (0, 1=w383:i16)
                        n186 = Boolean To (0,1)(Boolean=w390) -> (0, 1=w389:i16)
                        n187 = Boolean To (0,1)(Boolean=w394) -> (0, 1=w393:i16)
                        n188 = Boolean To (0,1)(Boolean=w388) -> (0, 1=w387:i16)
                        n189 = Boolean To (0,1)(Boolean=w392) -> (0, 1=w391:i16)
                        n190 = Boolean To (0,1)(Boolean=w386) -> (0, 1=w385:i16)
                        n191 = Unbundle By Name(w318) -> ("Bay 5 Parameters.optimize_temp"=w378:bool)
                        n192 = Unbundle By Name(w318) -> ("Bay 5 Parameters.optimize_tau"=w376:bool)
                        n193 = Index Array(array=w333, index=5) -> (element=w331:string)
                        n194 = Boolean To (0,1)(Boolean=w378) -> (0, 1=w377:i16)
                        n195 = Boolean To (0,1)(Boolean=w376) -> (0, 1=w375:i16)
                        n196 = Build Array(w393, w391, w389, w387, w385, w383, w381, w379, w377, w375) -> (w374:i16[])
                        n197 = Unbundle By Name(w318) -> ("Bay 1 Parameters.Temperature Params"=w371:dbl[])
                        n198 = Unbundle By Name(w318) -> ("Bay 2 Parameters.Temperature Params"=w370:dbl[])
                        n199 = Unbundle By Name(w318) -> ("Bay 2 Parameters.Resisdence time params"=w365:dbl[])
                        n200 = Unbundle By Name(w318) -> ("Bay 3 Parameters.Temperature Params"=w369:dbl[])
                        n201 = Unbundle By Name(w318) -> ("Bay 3 Parameters.Resisdence time params"=w364:dbl[])
                        n202 = Unbundle By Name(w318) -> ("Bay 4 Parameters.Temperature Params"=w368:dbl[])
                        n203 = Unbundle By Name(w318) -> ("Bay 4 Parameters.Resisdence time params"=w363:dbl[])
                        n204 = Unbundle By Name(w318) -> ("Bay 5 Parameters.Temperature Params"=w367:dbl[])
                        n205 = Unbundle By Name(w318) -> ("Bay 5 Parameters.Resisdence time params"=w362:dbl[])
                        n206 = Unbundle By Name(w318) -> ("Bay 1 Parameters.pump params 2"=w317:dbl[])
                        n207 = Unbundle By Name(w318) -> ("Bay 1 Parameters.pump params 1"=w366:dbl[])
                        n208 = Unbundle By Name(w318) -> ("Bay 3 Parameters.pump_num_ratio"=w346:dbl)
                        n209 = Unbundle By Name(w318) -> ("Bay 4 Parameters.pump_num_ratio"=w343:dbl)
                        n210 = Unbundle By Name(w318) -> ("Bay 5 Parameters.pump_num_ratio"=w340:dbl)
                        n211 = Unbundle By Name(w318) -> ("Bay 2 Parameters.pump_num_ratio"=w349:dbl)
                        n212 = Unbundle By Name(w318) -> ("Bay 4 Parameters.pump_at_ratio"=w345:bool)
                        n213 = Boolean To (0,1)(Boolean=w345) -> (0, 1=w344:i16)
                        n214 = Unbundle By Name(w318) -> ("Bay 3 Parameters.pump_at_ratio"=w348:bool)
                        n215 = Boolean To (0,1)(Boolean=w348) -> (0, 1=w347:i16)
                        n216 = Unbundle By Name(w318) -> ("Bay 5 Parameters.pump_at_ratio"=w342:bool)
                        n217 = Boolean To (0,1)(Boolean=w342) -> (0, 1=w341:i16)
                        n218 = Unbundle By Name(w318) -> ("Bay 2 Parameters.pump_at_ratio"=w351:bool)
                        n219 = Boolean To (0,1)(Boolean=w351) -> (0, 1=w350:i16)
                        n220 = script code="length_reactor1 = 188;%cm\nsystem_error = 0;\nlength_reactor2 = 99; %cm\nlength_bypass = 10;%cm\nnumPeaks = 1;\nstart_phase_time = 1;\nis_redo_exp = 0;\nFvalues = [];\nHPLC_Area = [];\ntube_diameters = [.01, .02, .03, .04];\nD1 = tube_diameters(tube_id(1) +1); D1 = D1*2.54;\nD2 = tube_diameters(tube_id(2) +1); D2 = D2*2.54;\nD3 = tube_diameters(tube_id(3) +1); D3 = D3*2.54;\nD4 = tube_diameters(tube_id(4) +1); D4 = D4*2.54;\nD5 = tube_diameters(tube_id(5) +1); D5 = D5*2.54;\nT1_span = [1 1]; T2_span = [1 1]; T3_span = [1 1]; T4_span = [1 1]; T5_span = [1 1];\n p1_span =  [1 1]; p2_span =  [1 1]; p3_span =  [1 1]; p4_span =  [1 1]; p5_span =  [1 1];  p6_span =  [1 1];\nOpt_params = [0 0 0 0 0 0 0 0 0 0 0];\nopt_ctr = 0;ncall = 100;\nrecord_data = true;\nT1_SP = 23; T2_SP = 23; T3_SP = 23; T4_SP = 23; T5_SP = 23;\nno_errors = 1;\nP1 = 0; P2 =0; P3 = 0; P4 = 0; P5 = 0; P6 = 0;\nis_first_set_of_exp = true;\nerror_message = 'System has no errors to report';\n%addpath(genpath('C:\\Users\\HPLC\\Dropbox (MIT)\\multistep_optimization'))\naddpath(genpath('C:\\Users\\HPLC\\Dropbox (MIT)\\MoD Files\\MATLAB'))\nallMSData = [];\nallHPLCData = [];\nallHPLCFile = [];\nCurrExp = 1;\nif Continue\n   load(matlabsavefile);\nelse\nx = []\n   IRSteadystate = 0;\n   ProductVec = [];\n   TwopointbaselineProductVec=[];\nend\nall_MSData = [];\n% ****************************************************************************************************\nif Bay1 == 1\n    %1.05m reactor\n     Vr1 = length_reactor1*D1^2/4*3.14159*1000;\n     if  Optimize_params(1)\n       % if choice is made to optimize temperature\n        if T1_params(2) < T1_params(3)\n             T1_span = [T1_params(2) ,  T1_params(3)];\n              Opt_params(1) = 1;\n         else\n            no_errors = 0;\n            error_message = 'Lower bound of temperature must be lower than upper bound';\n        end\n    else\n       %  if choice is made to not optimize temperature\n        T1_SP = T1_params(1);  \n    end\n\n    if Optimize_params(2)\n       % if user wants to optimize flowrates\n        if pump1_params(2) < pump1_params(3)\n             p1_span = [pump1_params(2) ,  pump1_params(3)];\n             p1_span = p1_span;\n             Opt_params(6) = 1; Opt_params(7) = 1;\n         else\n            no_errors = 0;\n            error_message = 'Lower bound of flowrate 1 must be lower than upper bound';\n        end\n         if pump2_params(2) < pump2_params(3)\n             p2_span = [pump2_params(2) ,  pump2_params(3)];\n             p2_span = p2_span;\n             Opt_params(6) = 1; Opt_params(7) = 1;\n         else\n            no_errors = 0;\n            error_message = 'Lower bound of flowrate 2 must be lower than upper bound';\n        end \n    else\n       if use_flowrate1\n            if P1_setrate < 0 || P2_setrate < 0\n               no_errors = 0;\n               error_message = 'Pump set flowrates can not be negative';\n            else\n               P1 = P1_setrate;\n               P2 = P1_setrate;\n            end\n       else\n            if pump1_params(1) > 0\n               P1 = pump1_params(1);\n            elseif not(isempty(pump1_chem))\n               no_errors = 0;\n               error_message = 'Bay1 Pump 1 setpoint must be greater than zero';\n            end\n             if pump2_params(1) > 0\n               P2 = pump2_params(1);\n            elseif not(isempty(pump2_chem))\n               no_errors = 0;\n               error_message = 'Bay1 Pump 2 setpoint must be greater than zero';\n            end\n       end\n    end\nelseif Bay1 == 0\n    % .1m bypass\n    Vr1 =length_bypass*D1^2/4*3.14159*1000;\n    if Optimize_params(1)\n          no_errors = 0;\n          error_message = 'Can not optimize temperature on bypass ';\n    end\n\n    if Optimize_params(2)\n       % if user wants to optimize residence time\n        if pump1_params(2) < pump1_params(3)\n             p1_span = [pump1_params(2) ,  pump1_params(3)];\n             p1_span = p1_span;\n             Opt_params(6) = 1; Opt_params(7) = 1;\n         else\n            no_errors = 0;\n            error_message = 'Lower bound of pump 1 must be lower than upper bound';\n        end\n       if pump2_params(2) < pump2_params(3)\n             p2_span = [pump2_params(2) ,  pump2_params(3)];\n             p2_span = p2_span;\n             Opt_params(6) = 1; Opt_params(7) = 1;\n         else\n            no_errors = 0;\n            error_message = 'Lower bound of pump 2 must be lower than upper bound';\n        end\n    else\n       if use_flowrate1\n            if P1_setrate < 0 || P2_setrate < 0\n               no_errors = 0;\n               error_message = 'Pump set flowrates can not be negative';\n            else\n               P1 = P1_setrate;\n               P2 = P2_setrate;\n            end\n       else\n            if pump1_params(1) > 0\n               P1 = pump1_params(1);\n            elseif not(isempty(pump1_chem))\n               no_errors = 0;\n               error_message = 'Bay 1 Pump 2 setpoint must be greater than zero';\n            end\n           if pump2_params(1) > 0\n               P2 = pump2_params(1);\n            elseif not(isempty(pump2_chem))\n               no_errors = 0;\n               error_message = 'Bay 1 Pump 2 setpoint must be greater than zero';\n            end\n       end\n    end\nelse\n    %separator\n    Vr1 = 1000;\n    if use_flowrate1\n        P1 = P1_setrate;\n        P2 = P2_setrate;\n    else \n        if not(isempty(pump1_chem))\n           P1 = 200;\n        end\n        if not(isempty(pump2_chem))\n           P2 = 200;\n        end\n    end\n    \nend\n\n% ****************************************************************************************************\n\n   if Bay2 == 1 \n   %1.05m reactor\n     Vr2 =length_reactor1*D2^2/4*3.14159*1000;\n     if  Optimize_params(3)\n       % if choice is made to optimize temperature\n        if T2_params(2) < T2_params(3)\n             T2_span = [T2_params(2) ,  T2_params(3)];\n             Opt_params(2) = 1;\n         else\n            no_errors = 0;\n            error_message = 'Lower bound of temperature must be lower than upper bound';\n        end\n    else\n       %  if choice is made to not optimize temperature\n        T2_SP = T2_params(1);  \n    end\n\n    if Optimize_params(4)\n       % if user wants to optimize residence time\n        if pump3_params(2) < pump3_params(3)\n             p3_span = [pump3_params(2) ,  pump3_params(3)];\n             p3_span = p3_span;\n             Opt_params(8) = 1;\n         else\n            no_errors = 0;\n            error_message = 'Lower bound of pump 3 must be lower than upper bound';\n        end\n    else\n       if use_flowrate2\n            if P3_setrate < 0\n               no_errors = 0;\n               error_message = 'Pump set flowrates can not be negative';\n            else\n               P3 = P3_setrate;\n            end\n       elseif Bay2_ratio\n            P3 = Bay2_pump_ratio*(P1); % changed from Bay2_pump_ratio*(P1+P2); \n       else\n            if pump3_params(1) > 0\n               P3 = pump3_params(1);\n            elseif not(isempty(pump3_chem))\n               no_errors = 0;\n               error_message = 'Bay 2 Pump 3 flowrate setpoint must be greater than zero';\n            end\n       end\n    end\nelseif Bay2 == 0\n    % .1m bypass\n    Vr2 =length_bypass*D2^2/4*3.14159*1000;\n    if Optimize_params(3)\n          no_errors = 0;\n          error_message = 'Can not optimize temperature on bypass ';\n    end\n\n    if Optimize_params(4)\n       % if user wants to optimize residence time\n        if pump3_params(2) < pump3_params(3)\n             p3_span = [pump3_params(2) ,  pump3_params(3)];\n             p3_span = p3_span;\n             Opt_params(8) = 1;\n         else\n            no_errors = 0;\n            error_message = 'Lower bound of resisdence time must be lower than upper bound';\n        end\n    else\n       if use_flowrate2\n            if P3_setrate < 0\n               no_errors = 0;\n               error_message = 'Pump set flowrates can not be negative';\n            else\n               P3 = P3_setrate;\n            end\n      elseif Bay2_ratio\n           P3 = Bay2_pump_ratio*(P1); % changed from Bay2_pump_ratio*(P1+P2); \n       else\n            if pump3_params(1) > 0\n               P3 = pump3_params(1);\n            elseif not(isempty(pump3_chem))\n               no_errors = 0;\n               error_message = 'Bay 2 Pump 3 setpoint must be greater than zero';\n            end\n       end\n    end\n   else\n    %separator\n    Vr2 = 1000;\n    if Optimize_params(4)\n       % if user wants to optimize residence time\n        if pump3_params(2) < pump3_params(3)\n             p3_span = [pump3_params(2) ,  pump3_params(3)];\n             p3_span = p3_span;\n             Opt_params(8) = 1;\n         else\n            no_errors = 0;\n            error_message = 'Lower bound of pump flowrate must be lower than upper bound';\n        end\n    else\n       if use_flowrate2\n           P3 = P3_setrate;\n       elseif Bay3_ratio\n           P3 = Bay2_pump_ratio*(P1); % changed from Bay2_pump_ratio*(P1+P2); \n       elseif not(isempty(pump3_chem))\n          P3 = 200;\n        end\n      end\n   end\n\n% ****************************************************************************************************\n\n  if Bay3 == 1 \n   %1.05m reactor\n     Vr3= length_reactor1*D3^2/4*3.14159*1000;\n     Vr3 = 1300;\n     if  Optimize_params(5)\n       % if choice is made to optimize temperature\n        if T3_params(2) < T3_params(3)\n             T3_span = [T3_params(2) ,  T3_params(3)];\n             Opt_params(3) = 1;\n         else\n            no_errors = 0;\n            error_message = 'Lower bound of temperature must be lower than upper bound';\n        end\n    else\n       %  if choice is made to not optimize temperature\n        T3_SP = T3_params(1);  \n    end\n\n    if Optimize_params(6)\n       % if user wants to optimize residence time\n        if pump4_params(2) < pump4_params(3)\n             p4_span = [pump4_params(2) ,  pump4_params(3)];\n             p4_span = p4_span;\n             Opt_params(9) = 1;\n         else\n            no_errors = 0;\n            error_message = 'Lower bound of pump 4 flowrate must be lower than upper bound';\n        end\n    else\n       if use_flowrate3\n            if P4_setrate < 0\n               no_errors = 0;\n               error_message = 'Pump set flowrates can not be negative';\n            else\n               P4 = P4_setrate;\n            end\n       elseif Bay3_ratio\n            P4= Bay3_pump_ratio*(P1+P2+P3);\n       else\n            if pump4_params(1) > 0\n               %Should a check be made whether or not tau1 > tau2\n                 P4 = pump4_params(1) ;\n            elseif not(isempty(pump4_chem))\n               no_errors = 0;\n               error_message = 'Bay 3 pump 4 setpoint must be greater than zero';\n            end\n       end\n    end\nelseif Bay3 == 0\n    % .1m bypass\n    Vr3 =length_bypass*D3^2/4*3.14159*1000;\n    if Optimize_params(5)\n          no_errors = 0;\n          error_message = 'Can not optimize temperature on bypass ';\n    end\n\n    if Optimize_params(6)\n       % if user wants to optimize residence time\n        if pump4_params(2) < pump4_params(3)\n             p4_span = [pump4_params(2) ,  pump4_params(3)];\n             p4_span = p4_span;\n             Opt_params(9) = 1;\n         else\n            no_errors = 0;\n            error_message = 'Lower bound of pump 4 setpoint must be lower than upper bound';\n        end\n    else\n       if use_flowrate3\n            if P4_setrate < 0\n               no_errors = 0;\n               error_message = 'Pump set flowrates can not be negative';\n            else\n               P4 = P4_setrate;\n            end\n       elseif Bay3_ratio\n            P4= Bay3_pump_ratio*(P1+P2+P3);\n       else\n            if pump4_params(1) > 0\n               P4 =pump4_params(1) ;\n            elseif not(isempty(pump4_chem))\n               no_errors = 0;\n               error_message = 'Bay 3 pump 4 setpoint must be greater than zero';\n            end\n       end\n    end\n   else\n    %separator\n      Vr3 = 1000;\n      if Optimize_params(6)\n       % if user wants to optimize residence time\n        if pump4_params(2) < pump4_params(3)\n             p4_span = [pump4_params(2) ,  pump4_params(3)];\n             p4_span = p4_span;\n             Opt_params(9) = 1;\n         else\n            no_errors = 0;\n            error_message = 'Lower bound of pump 4 flowrate must be lower than upper bound';\n        end\n     else\n        if use_flowrate3\n           P4 = P4_setrate;\n        elseif Bay3_ratio\n            P4= Bay3_pump_ratio*(P1+P2+P3);\n        elseif not(isempty(pump4_chem))\n          P4 = 200;\n        end\n      end\n   end\n\n% ****************************************************************************************************\n\n   if Bay4 == 1 \n   %1.05m reactor\n     Vr4 = length_reactor2*D4^2/4*3.14159*1000;\n     if  Optimize_params(7)\n       % if choice is made to optimize temperature\n        if T4_params(2) < T4_params(3)\n             T4_span = [T4_params(2) ,  T4_params(3)];\n              Opt_params(4) = 1;\n         else\n            no_errors = 0;\n            error_message = 'Lower bound of temperature must be lower than upper bound';\n        end\n    else\n       %  if choice is made to not optimize temperature\n        T4_SP = T4_params(1);  \n    end\n\n    if Optimize_params(8)\n       % if user wants to optimize residence time\n        if pump5_params(2) < pump5_params(3)\n             p5_span = [pump5_params(2) ,  pump5_params(3)];\n             p5_span = p5_span;\n            Opt_params(10) = 1;\n         else\n            no_errors = 0;\n            error_message = 'Lower bound of pump 5 flowrate must be lower than upper bound';\n        end\n    else\n       if use_flowrate4\n            if P5_setrate < 0\n               no_errors = 0;\n               error_message = 'Pump set flowrates can not be negative';\n            else\n               P5 = P5_setrate;\n            end\n       elseif Bay4_ratio\n            P5= Bay4_pump_ratio*(P1+P2+P3+P4);\n       else\n            if pump5_params(1) > 0\n               %Should a check be made whether or not tau4 > tau3\n                 P5 = pump5_params(1) ;\n            elseif not(isempty(pump5_chem))\n               no_errors = 0;\n               error_message = 'Bay 4 Pump 5 setpoint must be greater than zero';\n            end\n       end\n    end\nelseif Bay4 == 0\n    % .1m bypass\n    Vr4 =length_bypass*D4^2/4*3.14159*1000;\n    if Optimize_params(7)\n          no_errors = 0;\n          error_message = 'Can not optimize temperature on bypass ';\n    end\n\n    if Optimize_params(8)\n       % if user wants to optimize residence time\n        if pump5_params(2) < pump5_params(3)\n             p5_span = [pump5_params(2) ,  pump5_params(3)];\n             p5_span = p5_span;\n             Opt_params(10) = 1;\n         else\n            no_errors = 0;\n            error_message = 'Lower bound of resisdence time must be lower than upper bound';\n        end\n    else\n       if use_flowrate4\n            if P5_setrate < 0\n               no_errors = 0;\n               error_message = 'Pump set flowrates can not be negative';\n            else\n               P5 = P5_setrate;\n            end\n       elseif Bay4_ratio\n            P5= Bay4_pump_ratio*(P1+P2+P3+P4);\n       else\n            if pump5_params(1) > 0\n               P5 = pump5_params(1);\n            elseif not(isempty(pump5_chem))\n               no_errors = 0;\n               error_message = 'Bay 4 pump 5 setpoint must be greater than zero';\n            end\n       end\n    end\n   else\n    %separator\n      Vr4 = 1000;\n      if Optimize_params(8)\n       % if user wants to optimize residence time\n         if pump5_params(2) < pump5_params(3)\n             p5_span = [pump5_params(2) ,  pump5_params(3)];\n             p5_span = p5_span;\n             Opt_params(10) = 1;\n         else\n            no_errors = 0;\n            error_message = 'Lower bound of resisdence time must be lower than upper bound';\n         end\n       else\n           if use_flowrate4\n              P5 = P5_setrate;\n           elseif Bay4_ratio\n              P5= Bay4_pump_ratio*(P1+P2+P3+P4);\n           elseif not(isempty(pump5_chem))\n              P5 = 200;\n           end\n        end\n   end\n\n% ****************************************************************************************************\n\n  if Bay5 == 1 \n   %1.05m reactor\n     Vr5= length_reactor*D5^2/4*3.14159*1000;\n     if  Optimize_params(9)\n       % if choice is made to optimize temperature\n        if T5_params(2) < T5_params(3)\n             T5_span = [T5_params(2) ,  T5_params(3)];\n             Opt_params(5) = 1;\n         else\n            no_errors = 0;\n            error_message = 'Lower bound of temperature must be lower than upper bound';\n        end\n    else\n       %  if choice is made to not optimize temperature\n        T5_SP = T5_params(1);  \n    end\n\n    if Optimize_params(10)\n       % if user wants to optimize residence time\n        if pump6_params(2) < pump6_params(3)\n             p6_span = [pump6_params(2) ,  pump6_params(3)];\n             p6_span = p6_span;\n             Opt_params(11) = 1;\n         else\n            no_errors = 0;\n            error_message = 'Lower bound of pump 6 flowrate must be lower than upper bound';\n        end\n    else\n       if use_flowrate5\n            if P6_setrate < 0\n               no_errors = 0;\n               error_message = 'Pump set flowrates can not be negative';\n            else\n               P6 = P6_setrate;\n            end\n      elseif Bay5_ratio\n              P6= Bay5_pump_ratio*(P1+P2+P3+P4+P5);\n      else\n            if pump6_params(1) > 0\n               %Should a check be made whether or not tau1 > tau2\n                 P6 =pump6_params(1) ;\n            elseif not(isempty(pump6_chem))\n               no_errors = 0;\n               error_message = 'Bay 5 pump 6 setpoint must be greater than zero';\n            end\n       end\n    end\nelseif Bay5 == 0\n    % .1m bypass\n    Vr5 =length_bypass*D5^2/4*3.14159*1000;\n    if Optimize_params(9)\n          no_errors = 0;\n          error_message = 'Can not optimize temperature on bypass ';\n    end\n\n    if Optimize_params(10)\n       % if user wants to optimize residence time\n        if pump6_params(2) < pump6_params(3)\n             p6_span = [pump6_params(2) ,  pump6_params(3)];\n             p6_span = p6_span;\n             Opt_params(11) = 1;\n         else\n            no_errors = 0;\n            error_message = 'Lower bound of pump 6 must be lower than upper bound';\n        end\n    else\n       if use_flowrate5\n            if P6_setrate < 0\n               no_errors = 0;\n               error_message = 'Pump set flowrates can not be negative';\n            else\n               P6 = P6_setrate;\n            end\n      elseif Bay5_ratio\n              P6= Bay5_pump_ratio*(P1+P2+P3+P4+P5);\n       else\n            if pump6_params(1) > 0\n               P6 = pump6_params(1);\n            elseif not(isempty(pump6_chem))\n               no_errors = 0;\n               error_message = 'Bay 5 pump 6 setpoint must be greater than zero';\n            end\n       end\n    end\n   else\n    %separator\n      Vr5 = 1000;\n      if Optimize_params(10)\n       % if user wants to optimize residence time\n        if pump6_params(2) < pump6_params(3)\n             p6_span = [pump6_params(2) ,  pump6_params(3)];\n             p6_span = p6_span;\n             Opt_params(11) = 1;\n         else\n            no_errors = 0;\n            error_message = 'Lower bound of pump 6 must be lower than upper bound';\n        end\n      else\n         if use_flowrate5\n               P6 = P6_setrate;\n         elseif Bay5_ratio\n               P6= Bay5_pump_ratio*(P1+P2+P3+P4+P5);\n         elseif not(isempty(pump6_chem))\n              P6 = 200;\n         end\n      end\n   end\n\n% ****************************************************************************************************\n\n%Setup optimization\n\n   initialize_opt = 0;\n\n%*****************************************************************************************************\n% Setup excel and xml file writing\n\npath(path, pa);\nnumMSSig = 1;\n\n%Setup output excel file\n% Opening Excel file and inputing first peaks headers if needed\ntry\n  xlApp = actxGetRunningServer('Excel.Application');\ncatch ME\n  xlApp = actxserver('Excel.Application');\nend\n\nxlApp.DisplayAlerts = false; \nxlApp.Visible = false;\n\n%try\n   xlWorkbook = xlApp.workbooks.Open(xl_file, 0,false);\n   xlSheets = xlWorkbook.Sheets;\n   xlSheetNamesArray = cell(xlSheets.Count, 1);\n\n  for i = 1:xlSheets.Count\n     xlSheetNamesArray{i} = xlSheets.Item(i).Name;\n  end\n\n  [~, idx1] = ismember('Time_Series_Conditions', xlSheetNamesArray);\n  lastcol1 = xlcolumnletter(22);\n\n  [~, idx2] = ismember('MS Results', xlSheetNamesArray);\n  lastcol2 = xlcolumnletter(2);\n\n  [~, idx3] = ismember('System Setup', xlSheetNamesArray);\n  lastcol3 = xlcolumnletter(11);\n\n  [~, idx4] = ismember('HPLC Results', xlSheetNamesArray);\n  lastcol4 = xlcolumnletter(3);\n\n  [~, idx_ir_exp] = ismember('IR Results', xlSheetNamesArray);\n  IR_i= xlSheets.Item(idx_ir_exp).Range('A1').End('xlDown').Row ; \n  if IR_i == 1048576\n     IR_i = 2;\n  end\n \n  lastrow1 =  xlSheets.Item(idx1).Range('A1').End('xlDown').Row;\n  if lastrow1 == 1048576\n      lastrow1 = 2;\n  end\n\n  lastrow2 =  xlSheets.Item(idx2).Range('A1').End('xlDown').Row;\n  if lastrow2 == 1048576\n      lastrow2 = 2;\n  end\n\n   lastrow3= 2;\n\n    lastrow4=  xlSheets.Item(idx4).Range('A1').End('xlDown').Row;\n    if lastrow4 == 1048576\n       lastrow4 =2;\n    end\n\n%catch ME\n %   xlWorkbook = xlApp.Workbooks;\n %  xlWorkbook = invoke(xlWorkbook, 'Add');\n %   WS = xlWorkbook.Worksheets;\n %   row = num2str(1);\n %   temp_write = [Bay1, Bay2, Bay3, Bay4, Bay5, 1, Vr1, Vr2, Vr3, Vr4, Vr5];\n %   xlSheets.Item(idx3).Range(strcat('A',row,':',lastcol3,row)).Value2 =  temp_write;\n %   WS.Add([], WS.Item(WS.Count));\n %   WS.Item(WS.Count).Name = 'Time_Series_Conditions';\n %    WS.Add([], WS.Item(WS.Count));\n %    WS.Item(WS.Count).Name = 'MS Results';\n %   WS.Add([], WS.Item(WS.Count));\n %    WS.Item(WS.Count).Name = 'System Setup';\n %   WS.Add([], WS.Item(WS.Count));\n %    WS.Item(WS.Count).Name = 'HPLC Results';\n%end\n\nload('C:\\Users\\HPLC\\Dropbox (MIT)\\MoD Files\\MATLAB\\IR_Pks.mat');\n\ntemp_write = [Bay1, Bay2, Bay3, Bay4, Bay5, 1, Vr1, Vr2, Vr3, Vr4, Vr5];\nlastrowStr3 = num2str(lastrow3);\nxlSheets.Item(idx3).Range(strcat('A',lastrowStr3,':',lastcol3,lastrowStr3)).Value2 =  temp_write;\nlastrow3 = lastrow3 +1;\n\ntemp_write = {pump1_chem, pump2_chem, pump3_chem, pump4_chem, pump5_chem, pump6_chem};\nlastrowStr3 = num2str(6);\nxlSheets.Item(idx3).Range(strcat('B',lastrowStr3,':','G',lastrowStr3)).Value2 =  temp_write;\n\nlastrowStr3 = num2str(8);\nxlSheets.Item(idx3).Range(strcat('B',lastrowStr3,':','G',lastrowStr3)).Value2 = Pump_concen;\n\n\n\n%***************************************************************************************************\n\nredo = false;\nncall = ncall_in;"("Bay1"=w420, "Bay2"=w419, "Bay3"=w418, "Bay4"=w417, "Bay5"=w416, "tube_id"=w415, "use_flowrate1"=w402, "P1_setrate"=w414, "P2_setrate"=w413, "P3_setrate"=w412, "P4_setrate"=w411, "P5_setrate"=w410, "P6_setrate"=w409, "use_flowrate2"=w352, "use_flowrate3"=w399, "use_flowrate4"=w398, "use_flowrate5"=w395, "Optimize_params"=w374, "T1_params"=w371, "T2_params"=w370, "T3_params"=w369, "T4_params"=w368, "T5_params"=w367, "pump1_params"=w366, "pump3_params"=w365, "pump4_params"=w364, "pump5_params"=w363, "pump6_params"=w362, "P1_P2_ratio"=w359, "xml_file"=w358, "xl_file"=w357, "pa"=w356, "Continue"=w354, "matlabsavefile"=w353, "Bay2_ratio"=w350, "Bay2_pump_ratio"=w349, "Bay3_ratio"=w347, "Bay3_pump_ratio"=w346, "Bay4_ratio"=w344, "Bay4_pump_ratio"=w343, "Bay5_ratio"=w341, "Bay5_pump_ratio"=w340, "pump1_chem"=w332, "pump6_chem"=w331, "pump5_chem"=w330, "pump4_chem"=w329, "pump3_chem"=w328, "pump2_chem"=w327, "Pump_concen"=w320, "ncall_in"=w319, "pump2_params"=w317) -> ("Vr1"=w408:dbl, "Vr2"=w407:dbl, "Vr3"=w406:dbl, "Vr4"=w405:dbl, "Vr5"=w404:dbl, "no_errors"=w373:dbl, "error_message"=w372:string)  [unwired: 1 in, 1 out]
                        n221 = Not Equal To 0?(x=w373) -> (x != 0?=w360:bool)
                        n222 = Not(x=w360) -> (.not. x?=w361:bool)
                        n223 = case shown="True" w361 {
                          tunnel: w372 -> [_ w421]
                          frame False {
                          }
                          frame True {
                            n224 = One Button Dialog(message=w421) -> ()  [unwired: 1 in, 1 out]
                          }
                        }
                      }
                    }
                    n225 = local read "Stop"() -> (w292:bool)
                    n226 = Or(x=w284, y=w292) -> (x .or. y?=w293:bool)
                    n227 = Wait (ms)(milliseconds to wait=u32 500) -> ()  [unwired: 1 out]
                  }
                  n228 = local write "Volume (ul) 1"(w278) -> ()
                  n229 = local write "Volume (ul) 2"(w277) -> ()
                  n230 = local write "Volume (ul) 3"(w276) -> ()
                  n231 = local write "Volume (ul) 4"(w275) -> ()
                  n232 = local write "Volume (ul) 5"(w274) -> ()
                }
                frame #2 {
                  n233 = local write "Setup Confirm 2"(w422) -> ()
                }
              }
            }
          }
        }
        frame #2 {
          # "Run Initial diagnostics"
        }
        frame #3 {
          # "Run System"
          n234 = while {
            tunnel: w424 -> [w1179]
            stop <- w1181 stop-if-true
            n235 = local read "Debug_run_button"() -> (w1176:bool)
            n236 = Not(x=w1176) -> (.not. x?=w1178:bool)
            n237 = local read "Temperature Control 1"() -> (w1175:bool)
            n238 = And(x=w1178, y=w1175) -> (x .and. y?=w1177:bool)
            n239 = case shown="True" w1177 {
              tunnel: w1179 -> [_ w1199]
              frame False {
                n240 = local write "Temp SS? 1"(TRUE ("Temp SS? 1")) -> ()
              }
              frame True {
                # "Bay 1 Temperature Controller"
                n241 = local read "Temperature SP 1"() -> (w1183:dbl)
                n242 = local read "Temperature 1"() -> (w1187:dbl)
                n243 = local read "SSR Duration 1"() -> (w1203:dbl)
                n244 = call-poly <vilib>:"PID Online Autotuning.vi"("setpoint"=w1183, "manipulated variable"=w1203, "autotuning parameters"=T7 {"type of controller"=enum."PID", "relay cycles"=3, "relay amplitude"=1.0, "control specifications"=enum."Normal", "PV noise level"=0.1} ("Autotuning Parameters R1"), "process variable"=w1187, "PID gains in"=T6 {"Proportional gain Kc"=0.38538, "Integral time Ti (sec)"=0.524375, "Derivative time Ti (sec)"=0.12585} ("PID gains 2")) -> ("setpoint out"=w1209:dbl, "process variable out"=w1208:dbl, "PID gains out"=w1205:T14)  [unwired: 6 in, 2 out]
                n245 = call <vilib>:"PID Autotuning (Temperature).vi"("desired temperature"=w1209, "measured temperature"=w1208, "plant parameters in"=w1205, "output range"=cluster{"output high":dbl, "output low":dbl} {"output high"=3.0, "output low"=-1.0} ("Output range")) -> ("output"=w1201:dbl)  [unwired: 12 in, 3 out]
                n246 = local write "SSR Duration 1"(w1201) -> ()
                n247 = Subtract(x=w1183, y=w1187) -> (x-y=w1194:dbl)
                n248 = Absolute Value(x=w1194) -> (abs(x)=w1197:dbl)
                n249 = Multiply(x=1000.0, y=w1201) -> (x*y=w1198:dbl)
                n250 = Greater Than 0?(x=w1198) -> (x > 0?=w1192:bool)
                n251 = Less Or Equal?(x=w1197, y=1.2) -> (x <= y?=w1195:bool)
                n252 = Greater?(x=w1183, y=w1187) -> (0:w1193:bool)
                n253 = And(x=w1192, y=w1193) -> (x .and. y?=w1190:bool)
                n254 = local write "Temp SS? 1"(w1195) -> ()
                n255 = Subtract(x=w1187, y=10.0) -> (x-y=w1188:dbl)
                n256 = Less?(x=w1188, y=w1183) -> (x < y?=w1191:bool)
                n257 = And(x=w1191, y=w1190) -> (x .and. y?=w1189:bool)
                n258 = case shown="True" w1189 {
                  tunnel: [errorcluster {"status"=FALSE, "code"=0, "source"=""} ("error out") w1221] -> _
                  tunnel: w1199 -> [w1214 w1223]
                  tunnel: 2 -> [_ w1222]
                  tunnel: [w1214 w1220] -> _
                  tunnel: w1198 -> [w1213 w1219]
                  tunnel: [0.0 w1218] -> w1185
                  tunnel: w1183 -> [_ w1217]
                  frame False {
                    n259 = Absolute Value(x=w1213) -> (abs(x)=w1215:dbl)
                    n260 = Wait (ms)(milliseconds to wait=w1215) -> ()  [unwired: 1 out]
                  }
                  frame True {
                    n261 = call "TurnOnRelayArduino.vi"("channel"=w1222, "duration"=w1219, "LINX Resource"=w1223) -> ("error out"=w1221:errorcluster, "LINX Resource Out"=w1220:T8)  [unwired: 7 in]
                    n262 = script code="tempdiff1= SP1 - T1;\nif tempdiff1 > 10\n  if slope1 < .01\n     temp_check1 = temp_check1 + 1;\n  else\n      temp_check1 =0;\n  end\nend\n\nif temp_check1 > 9\n  temp_error1 = 1\nend"("SP1"=w1217) -> ("temp_error1"=w1218:dbl)  [unwired: 1 in, 1 out]
                  }
                }
                n263 = Not Equal To 0?(x=w1185) -> (x != 0?=w1184:bool)
                n264 = case shown="True" w1184 {
                  frame False {
                  }
                  frame True {
                    n265 = local write "Error Message"("Bay 1 Temperature Heating Error") -> ()
                  }
                }
                n266 = case shown="True" w1184 {
                  tunnel: w1184 -> [_ w1211]
                  frame False {
                  }
                  frame True {
                    n267 = local write "Stop"(w1211) -> ()
                  }
                }
              }
            }
            n268 = Wait (ms)(milliseconds to wait=u32 400) -> ()  [unwired: 1 out]
            n269 = local read "Stop"() -> (w1181:bool)
          }
          n270 = local read "Bay Parameters"() -> (w427:T3)
          n271 = while {
            tunnel: w424 -> [w1130]
            stop <- w1132 stop-if-true
            n272 = local read "Debug_run_button"() -> (w1127:bool)
            n273 = Not(x=w1127) -> (.not. x?=w1129:bool)
            n274 = local read "Temperature Control 2"() -> (w1126:bool)
            n275 = And(x=w1129, y=w1126) -> (x .and. y?=w1128:bool)
            n276 = case shown="True" w1128 {
              tunnel: w1130 -> [_ w1153]
              frame False {
                n277 = local write "Temp SS? 2"(TRUE ("Temp SS? 2")) -> ()
              }
              frame True {
                # "Bay 2 Temperature Controller"
                n278 = local read "Temperature SP 2"() -> (w1135:dbl)
                n279 = local read "Temperature 2"() -> (w1138:dbl)
                n280 = local read "SSR Duration 2"() -> (w1157:dbl)
                n281 = call-poly <vilib>:"PID Online Autotuning.vi"("setpoint"=w1135, "manipulated variable"=w1157, "autotuning parameters"=T7 {"type of controller"=enum."PID", "relay cycles"=3, "relay amplitude"=1.0, "control specifications"=enum."Normal", "PV noise level"=0.1} ("Autotuning Parameters R1"), "process variable"=w1138, "PID gains in"=T6 {"Proportional gain Kc"=0.38538, "Integral time Ti (sec)"=0.524375, "Derivative time Ti (sec)"=0.12585} ("PID gains 2")) -> ("setpoint out"=w1155:dbl, "process variable out"=w1154:dbl, "PID gains out"=w1160:T14)  [unwired: 6 in, 2 out]
                n282 = call <vilib>:"PID Autotuning (Temperature).vi"("desired temperature"=w1155, "measured temperature"=w1154, "plant parameters in"=w1160, "output range"=cluster{"output high":dbl, "output low":dbl} {"output high"=3.0, "output low"=-1.0} ("Output range")) -> ("output"=w1149:dbl)  [unwired: 12 in, 3 out]
                n283 = local write "SSR Duration 2"(w1149) -> ()
                n284 = Greater?(x=w1135, y=w1138) -> (0:w1144:bool)
                n285 = Multiply(x=1000.0, y=w1149) -> (x*y=w1151:dbl)
                n286 = Greater Than 0?(x=w1151) -> (x > 0?=w1143:bool)
                n287 = And(x=w1143, y=w1144) -> (x .and. y?=w1141:bool)
                n288 = Subtract(x=w1135, y=w1138) -> (x-y=w1146:dbl)
                n289 = Absolute Value(x=w1146) -> (abs(x)=w1148:dbl)
                n290 = Subtract(x=w1138, y=10.0) -> (x-y=w1140:dbl)
                n291 = Less Or Equal?(x=w1148, y=1.2) -> (x <= y?=w1145:bool)
                n292 = local write "Temp SS? 2"(w1145) -> ()
                n293 = Less?(x=w1140, y=w1135) -> (x < y?=w1142:bool)
                n294 = And(x=w1142, y=w1141) -> (x .and. y?=w1137:bool)
                n295 = case shown="True" w1137 {
                  tunnel: [errorcluster {"status"=FALSE, "code"=0, "source"=""} ("error out") w1172] -> _
                  tunnel: w1153 -> [w1165 w1174]
                  tunnel: 3 -> [_ w1173]
                  tunnel: [w1165 w1171] -> _
                  tunnel: w1151 -> [w1164 w1170]
                  tunnel: [0.0 w1169] -> w1136
                  tunnel: w1135 -> [_ w1168]
                  frame False {
                    n296 = Absolute Value(x=w1164) -> (abs(x)=w1166:dbl)
                    n297 = Wait (ms)(milliseconds to wait=w1166) -> ()  [unwired: 1 out]
                  }
                  frame True {
                    n298 = call "TurnOnRelayArduino.vi"("channel"=w1173, "duration"=w1170, "LINX Resource"=w1174) -> ("error out"=w1172:errorcluster, "LINX Resource Out"=w1171:T8)  [unwired: 7 in]
                    n299 = script code="tempdiff2= SP2 - T2;\nif tempdiff2 > 10\n  if slope2 < .01\n     temp_check2 = temp_check2 + 1;\n  else\n      temp_check2 =0;\n  end\nend\n\nif temp_check2 > 9\n  temp_error2 = 1\nend"("SP2"=w1168) -> ("temp_error2"=w1169:dbl)  [unwired: 1 in, 1 out]
                  }
                }
                n300 = Not Equal To 0?(x=w1136) -> (x != 0?=w1134:bool)
                n301 = case shown="True" w1134 {
                  frame False {
                  }
                  frame True {
                    n302 = local write "Error Message"("Bay 2 Temperature Heating Error") -> ()
                  }
                }
                n303 = case shown="True" w1134 {
                  tunnel: w1134 -> [_ w1162]
                  frame False {
                  }
                  frame True {
                    n304 = local write "Stop"(w1162) -> ()
                  }
                }
              }
            }
            n305 = local read "Stop"() -> (w1132:bool)
            n306 = Wait (ms)(milliseconds to wait=u32 400) -> ()  [unwired: 1 out]
          }
          n307 = local read "Stop"() -> (w423:bool)
          n308 = Not(x=w423) -> (.not. x?=w426:bool)
          n309 = case shown="True" w426 {
            tunnel: w427 -> [_ w433]
            tunnel: w424 -> [_ w432]
            tunnel: w425 -> [_ w431]
            tunnel: w424 -> [_ w430]
            frame False {
            }
            frame True {
              n310 = while {
                tunnel: w432 -> [w447]
                tunnel: w433 -> [w446]
                tunnel: w431 -> [w438]
                tunnel: w430 -> [w437]
                i -> [w445]
                stop <- w439 stop-if-true
                n311 = local read "Debug_run_button"() -> (w449:bool)
                n312 = Wait (ms)(milliseconds to wait=u32 1000) -> ()  [unwired: 1 out]
                n313 = Increment(x=w445) -> (x+1=w434:i32)
                n314 = case shown="False" w449 {
                  tunnel: w447 -> [_ _]
                  tunnel: w445 -> [_ w976]
                  tunnel: w446 -> [_ _]
                  tunnel: [w454 w978] -> w435
                  tunnel: [w455 0.0] -> w441
                  tunnel: w438 -> [w453 _]
                  tunnel: w437 -> [w452 _]
                  frame False {
                    n315 = flat-sequence {
                      tunnel: w453 -> [w457]
                      tunnel: [w457] -> w451
                      tunnel: [w465] -> w455
                      tunnel: [200.0] -> w454
                      tunnel: w452 -> [w462]
                      tunnel: w451 -> [w463]
                      frame #0 {
                        n316 = local write "stop_xl_write"(FALSE ("stop_xl_write")) -> ()
                      }
                      frame #1 {
                        # "Increase flowrate of dilution stream"
                        # "Wait mixed stream reaches SL"
                        # "SNOBFIT"
                        # "Optimize"
                        # "Run Experimental Conditions"
                        # "Optimize/Synthesize"
                        n317 = local read "Stop"() -> (w459:bool)
                        n318 = Not(x=w459) -> (.not. x?=w458:bool)
                        n319 = case shown="True" w458 {
                          tunnel: [1.0 w481] -> w468
                          tunnel: [dbl[] [] w480] -> w461
                          tunnel: [0.0 w479] -> w460
                          frame False {
                          }
                          frame True {
                            n320 = script code="if not(system_error)\n\nif not(redo)\n    % snobfit\n    snobfit_labview_driver;\n\n    if opt_ctr == 2\n      new_x = x(req_ctr,:);\n      x_ind = 1;\n      \n      if Opt_params(1)\n         T1_SP = new_x(x_ind ); %'C\n         params_1(1) = new_x(x_ind);\n         x_ind  = x_ind  + 1;\n      end\n     if Opt_params(2)\n       T2_SP = new_x(x_ind ); %'C\n        params_1(3) = new_x(x_ind);\n       x_ind  = x_ind  + 1;\n     end\n     if Opt_params(3)\n       T3_SP = new_x(x_ind ); %'C\n       x_ind  = x_ind  + 1;\n    end\n     if Opt_params(4)\n       T4_SP = new_x(x_ind ); %'C\n       x_ind  = x_ind  + 1;\n    end\n     if Opt_params(5)\n       T5_SP = new_x(x_ind ); %'C\n       x_ind  = x_ind  + 1;\n    end\n    if Opt_params(6)\n        tau1 = Vr1/(new_x( x_ind) +new_x( x_ind+1) );\n        %new_x( x_ind) = tau1*60;\n        params_1(2) = new_x(x_ind);\n        P2 =new_x( x_ind+1); %ul/min\n        P1=new_x( x_ind); %ul/min\n        x_ind  = x_ind  + 2;\n    end\n     if Opt_params(8)\n        tau2= Vr2/(new_x( x_ind)+P1+P2);\n        %new_x( x_ind) = tau2*60;\n        params_1(4) = new_x(x_ind);\n        P3=new_x( x_ind); %ul/minP2 = Vr4/(tau4)*60/2;\n        x_ind  = x_ind  + 1;\n      % P2 = Vr4/(tau4)*60/2;\n     elseif Bay2_ratio && not(use_flowrate2)\n        P3= Bay2_pump_ratio*(P1+P2); %chnaged from  P3= Bay2_pump_ratio*(P1 + P2);\n      end\n    if Opt_params(9)\n      tau3 =Vr3/(new_x( x_ind)+P1+P2+P3);\n      P4=new_x( x_ind); %ul/min\n      P3= Bay2_pump_ratio*(P4); \n      x_ind  = x_ind  + 1;\n    elseif Bay3_ratio && not(use_flowrate3)\n        P4= Bay3_pump_ratio*(P1+P2 +P3);\n    end\n    if Opt_params(10)\n      tau4 = Vr4/(new_x( x_ind)+P1+P2+P3+P4);\n      P5=new_x( x_ind) ; %ul/min\n       x_ind  = x_ind  + 1;\n    elseif Bay4_ratio && not(use_flowrate4)\n        P5= Bay4_pump_ratio*(P1+P2 +P3 +P4);\n    end\n    if Opt_params(11)\n      tau5 = Vr5/(new_x( x_ind)+P1+P2+P3+P4+P5);\n      %new_x( x_ind) = tau5*60;\n      P6=new_x( x_ind) ; %ul/min\n      x_ind  = x_ind  + 1;\n    elseif Bay5_ratio && not(use_flowrate5)\n        P6= Bay5_pump_ratio*(P1+P2 +P3 +P4 +P4 +P5);\n    end\n    %---------  \n end\n\n   P1=P1*2; P2 =P2*2; P3=P3*2; P4=P4*2; P5=P5*2; P6=P6*2;\n   Conditions_Array = [P1 P2 P3 P4 P5 P6 T1_SP T2_SP T3_SP T4_SP T5_SP];\n   if opt_ctr == 2\n        opt_ctr = 1;\n   else\n       opt_ctr = 2\n   end\nelse\n   opt_ctr =1;\n   redo = false;\n   is_redo_exp = 1;\n   if req_ctr ~= req_tot\n       req_ctr = req_ctr - 1;\n   end\n   CurrExp = CurrExp - 1;\n   ncall0 = ncall0 - 1;\n end\n\nend\n\nP_tot = P1 + P2 + P3 + P4 + P5 + P6 ;"() -> ("Conditions_Array"=w480:dbl[], "opt_ctr"=w481:dbl, "P_tot"=w479:dbl)  [unwired: 1 in, 1 out]
                          }
                        }
                        "P_tot" <- w460
                        n321 = local read "COMM Port :: Milligat Pumps"() -> (w469:refnum<visa-resource-name>)
                        n322 = Equal?(x=w468, y=1.0) -> (x = y?=w466:bool)
                        n323 = flat-sequence {
                          tunnel: w461 -> [w931]
                          frame #0 {
                            # "Start recording data"
                            n324 = Index Array(array=w931, index=5) -> (element=w948:dbl)
                            n325 = Index Array(array=w931, index=0) -> (element=w940:dbl)
                            n326 = Index Array(array=w931, index=1) -> (element=w941:dbl)
                            n327 = Index Array(array=w931, index=2) -> (element=w946:dbl)
                            n328 = Index Array(array=w931, index=3) -> (element=w945:dbl)
                            n329 = Index Array(array=w931, index=4) -> (element=w947:dbl)
                            n330 = local read "Volume (ul) 3"() -> (w918:dbl)
                            n331 = local read "Volume (ul) 5"() -> (w916:dbl)
                            n332 = local read "Volume (ul) 4"() -> (w917:dbl)
                            n333 = local read "Volume (ul) 2"() -> (w919:dbl)
                            n334 = local read "Volume (ul) 1"() -> (w920:dbl)
                            n335 = Add(x=w940, y=w941) -> (x+y=w929:dbl)
                            n336 = Add(x=w929, y=w946) -> (x+y=w927:dbl)
                            n337 = Add(x=w927, y=w945) -> (x+y=w925:dbl)
                            n338 = Add(x=w925, y=w947) -> (x+y=w922:dbl)
                            n339 = Add(x=w922, y=w948) -> (x+y=w924:dbl)
                            n340 = local write "Pump setpoint(ul/min) 2"(w941) -> ()
                            n341 = local write "Pump setpoint(ul/min) 4"(w946) -> ()
                            n342 = local write "Pump setpoint(ul/min) 5"(w947) -> ()
                            n343 = Not Equal To 0?(x=w929) -> (x != 0?=w930:bool)
                            n344 = local write "Pump setpoint(ul/min) 3"(w945) -> ()
                            n345 = local write "Pump setpoint(ul/min) 6"(w948) -> ()
                            n346 = local write "Pump setpoint(ul/min) 1"(w940) -> ()
                            n347 = Not Equal To 0?(x=w924) -> (x != 0?=w921:bool)
                            n348 = Not Equal To 0?(x=w925) -> (x != 0?=w926:bool)
                            n349 = Not Equal To 0?(x=w922) -> (x != 0?=w923:bool)
                            n350 = Not Equal To 0?(x=w927) -> (x != 0?=w928:bool)
                            n351 = case shown="False" w928 {
                              tunnel: w927 -> [_ w964]
                              tunnel: [0.0 w963] -> w939
                              tunnel: w919 -> [_ w962]
                              frame False {
                              }
                              frame True {
                                n352 = Divide(x=w962, y=w964) -> (x/y=w963:dbl)
                              }
                            }
                            n353 = case shown="True" w921 {
                              tunnel: w924 -> [_ w956]
                              tunnel: [0.0 w955] -> w944
                              tunnel: w916 -> [_ w954]
                              frame False {
                              }
                              frame True {
                                n354 = Divide(x=w954, y=w956) -> (x/y=w955:dbl)
                              }
                            }
                            n355 = case shown="True" w926 {
                              tunnel: [0.0 w960] -> w942
                              tunnel: w925 -> [_ w959]
                              tunnel: w918 -> [_ w958]
                              frame False {
                              }
                              frame True {
                                n356 = Divide(x=w958, y=w959) -> (x/y=w960:dbl)
                              }
                            }
                            n357 = case shown="True" w930 {
                              tunnel: w929 -> [_ w970]
                              tunnel: [0.0 w967] -> w938
                              tunnel: w920 -> [_ w969]
                              frame False {
                              }
                              frame True {
                                n358 = Divide(x=w969, y=w970) -> (x/y=w968:dbl)
                                n359 = Multiply(x=w968, y=0.0) -> (x*y=w967:dbl)
                              }
                            }
                            n360 = case shown="True" w923 {
                              tunnel: w922 -> [_ w952]
                              tunnel: [0.0 w951] -> w943
                              tunnel: w917 -> [_ w950]
                              frame False {
                              }
                              frame True {
                                n361 = Divide(x=w950, y=w952) -> (x/y=w951:dbl)
                              }
                            }
                            n362 = local write "tau 2"(w939) -> ()
                            n363 = local write "tau 3"(w942) -> ()
                            n364 = local write "tau 4"(w943) -> ()
                            n365 = local write "tau 5"(w944) -> ()
                            n366 = local write "tau 1"(w938) -> ()
                          }
                        }
                        n367 = flat-sequence {
                          tunnel: w469 -> [w485]
                          tunnel: w461 -> [w484]
                          tunnel: w466 -> [w483]
                          tunnel: [w483] -> w475
                          tunnel: w463 -> [w482]
                          tunnel: w475 -> [w616]
                          tunnel: [w616] -> w474
                          tunnel: w474 -> [w636]
                          tunnel: [w634] -> w473
                          tunnel: w462 -> [w670]
                          tunnel: w461 -> [w669]
                          tunnel: w473 -> [w668]
                          tunnel: [w863] -> w472
                          tunnel: w472 -> [w870]
                          tunnel: [w870] -> w471
                          tunnel: w471 -> [w878]
                          tunnel: [w878] -> w470
                          tunnel: [w915] -> w465
                          tunnel: w470 -> [w915]
                          frame #0 {
                            # "Setup pump flowrates and temperature setpoints"
                            n368 = stacked-sequence {
                              tunnel: w485 -> [w502 _ _ _ _]
                              tunnel: w485 -> [_ w541 _ _ _]
                              tunnel: w485 -> [_ _ w562 _ _]
                              tunnel: w485 -> [_ _ _ w583 _]
                              tunnel: w485 -> [_ _ _ _ w606]
                              tunnel: w484 -> [w499 w539 w560 w581 w601]
                              tunnel: w483 -> [w488 w531 w552 w573 w594]
                              tunnel: w482 -> [w486 _ _ _ _]
                              frame #0 {
                                # "Bay 1"
                                n369 = local read "Syringe_pump?"() -> (w487:bool)
                                n370 = Index Array(array=w499, index=0) -> (element=w497:dbl)
                                n371 = local read "Bay 1"() -> (w504:u16)
                                n372 = Index Array(array=w499, index=1) -> (element=w496:dbl)
                                n373 = Index Array(array=w499, index=6) -> (element=w495:dbl)
                                n374 = script code="MATLAB script"("P1"=w497, "P2"=w496, "T1_SP"=w495) -> ()  [unwired: 1 in, 1 out]
                                n375 = Greater Than 0?(x=w497) -> (x > 0?=w494:bool)
                                n376 = And(x=w494, y=w488) -> (x .and. y?=w493:bool)
                                n377 = Greater Than 0?(x=w496) -> (x > 0?=w492:bool)
                                n378 = Equal?(x=w504, y=u16 1) -> (x = y?=w490:bool)
                                n379 = And(x=w492, y=w488) -> (x .and. y?=w491:bool)
                                n380 = And(x=w490, y=w488) -> (x .and. y?=w489:bool)
                                n381 = case shown="True" w487 {
                                tunnel: w502 -> [w507 _]
                                tunnel: w496 -> [w506 w514]
                                tunnel: w491 -> [w505 w515]
                                tunnel: w486 -> [_ w513]
                                frame False {
                                n382 = case shown="True" w505 {
                                tunnel: w507 -> [w509 w511]
                                tunnel: w506 -> [_ w510]
                                frame False {
                                n383 = call "PumpStop.vi"("Pump Address"="j", "Pump COMM Port"=w509) -> ()  [unwired: 9 in, 1 out]
                                }
                                frame True {
                                n384 = call "PumpDispense.vi"("Flowrate(ul/min)"=w510, "Pump Address"="j", "Pump COMM Port"=w511) -> ()  [unwired: 7 in, 2 out]
                                }
                                }
                                }
                                frame True {
                                n385 = case shown="False" w515 {
                                tunnel: w514 -> [_ w521]
                                tunnel: w513 -> [w516 w522]
                                frame False {
                                n386 = call <instrlib>:"Stop Pump.vi"("VISA resource name"=w516) -> ()  [unwired: 9 in, 2 out]
                                }
                                frame True {
                                w517 = u16 0 items=["Infuse", "Withdraw"] ("Run Direction (0:Infuse)")
                                w518 = u32 4 items=["milliliters per hour (ml/hr)", "milliliters per minute (ml/min)", "milliliters per second (ml/sec)", "microliters per hour (ul/hr)", "microliters per minute (ul/min)", "microliters per second (ul/sec)", "nanoliters per hour (nl/hr)", "nanoliters per minute (nl/min)", "nanoliters per second (nl/sec)", "picoliters per hour (pl/hr)", "picoliters per minute (pl/min)", "picoliters per second (pl/sec)"] ("Flow Rate Units (1:ml/min)")
                                w519 = u16 0 items=["Infuse", "Withdraw"] ("Pump Direction (0:Infuse)")
                                n387 = call <instrlib>:"Configure Flow Rate & Direction.vi"("VISA resource name"=w522, "Pump Direction (0:Infuse)"=w519, "Flow Rate (5.00)"=w521, "Flow Rate Units (1:ml/min)"=w518) -> ("VISA resource name out"=w520:refnum<visa-resource-name>)  [unwired: 10 in, 1 out]
                                n388 = call <instrlib>:"Start Pump.vi"("Run Direction (0:Infuse)"=w517, "VISA resource name"=w520) -> ()  [unwired: 8 in, 2 out]
                                }
                                }
                                }
                                }
                                n389 = case shown="True" w493 {
                                tunnel: w502 -> [w526 w529]
                                tunnel: w497 -> [_ w528]
                                frame False {
                                n390 = call "PumpStop.vi"("Pump Address"="g", "Pump COMM Port"=w526) -> ()  [unwired: 9 in, 1 out]
                                }
                                frame True {
                                # "switched j and g"
                                n391 = call "PumpDispense.vi"("Flowrate(ul/min)"=w528, "Pump Address"="g", "Pump COMM Port"=w529) -> ()  [unwired: 7 in, 2 out]
                                }
                                }
                                n392 = case shown="True" w489 {
                                tunnel: w495 -> [_ w525]
                                frame False {
                                n393 = local write "Temperature Control 1"(FALSE) -> ()
                                }
                                frame True {
                                n394 = local write "Temperature SP 1"(w525) -> ()
                                n395 = local write "Temperature Control 1"(TRUE ("Temperature Control 1")) -> ()
                                }
                                }
                              }
                              frame #1 {
                                # "Bay 2"
                                n396 = Index Array(array=w539, index=2) -> (element=w536:dbl)
                                n397 = Index Array(array=w539, index=7) -> (element=w537:dbl)
                                n398 = script code="MATLAB script"("T2_SP"=w537, "P3"=w536) -> ()  [unwired: 1 in, 1 out]
                                n399 = local read "Bay 2"() -> (w542:u16)
                                n400 = Equal?(x=w542, y=u16 1) -> (x = y?=w535:bool)
                                n401 = Greater Than 0?(x=w536) -> (x > 0?=w533:bool)
                                n402 = And(x=w535, y=w531) -> (x .and. y?=w534:bool)
                                n403 = And(x=w533, y=w531) -> (x .and. y?=w532:bool)
                                n404 = case shown="True" w534 {
                                tunnel: w537 -> [_ w550]
                                frame False {
                                n405 = local write "Temperature Control 2"(FALSE) -> ()
                                }
                                frame True {
                                n406 = local write "Temperature Control 2"(TRUE ("Temperature Control 2")) -> ()
                                n407 = local write "Temperature SP 2"(w550) -> ()
                                }
                                }
                                n408 = case shown="True" w532 {
                                tunnel: w536 -> [_ w546]
                                tunnel: w541 -> [w545 w547]
                                frame False {
                                n409 = call "PumpStop.vi"("Pump Address"="i", "Pump COMM Port"=w545) -> ()  [unwired: 9 in, 1 out]
                                }
                                frame True {
                                n410 = call "PumpDispense.vi"("Flowrate(ul/min)"=w546, "Pump Address"="i", "Pump COMM Port"=w547) -> ()  [unwired: 7 in, 2 out]
                                }
                                }
                              }
                              frame #2 {
                                # "Bay 3"
                                n411 = Index Array(array=w560, index=3) -> (element=w557:dbl)
                                n412 = local read "Bay 3"() -> (w564:u16)
                                n413 = Not Equal To 0?(x=w557) -> (x != 0?=w556:bool)
                                n414 = Index Array(array=w560, index=8) -> (element=w558:dbl)
                                n415 = script code="MATLAB script"("T3_SP"=w558, "P4"=w557) -> ()  [unwired: 1 in, 1 out]
                                n416 = Equal?(x=w564, y=u16 1) -> (x = y?=w554:bool)
                                n417 = And(x=w554, y=w552) -> (x .and. y?=w553:bool)
                                n418 = And(x=w556, y=w552) -> (x .and. y?=w555:bool)
                                n419 = case shown="True" w553 {
                                tunnel: w558 -> [_ w571]
                                frame False {
                                n420 = local write "Temperature Control 3"(FALSE) -> ()
                                }
                                frame True {
                                n421 = local write "Temperature Control 3"(TRUE ("Temperature Control 3")) -> ()
                                n422 = local write "Temperature SP 3"(w571) -> ()
                                }
                                }
                                n423 = case shown="False" w555 {
                                tunnel: w557 -> [_ w567]
                                tunnel: w562 -> [w565 w569]
                                frame False {
                                n424 = call "PumpStop.vi"("Pump Address"="e", "Pump COMM Port"=w565) -> ()  [unwired: 9 in, 1 out]
                                }
                                frame True {
                                n425 = call "PumpDispense.vi"("Flowrate(ul/min)"=w567, "Pump Address"="e", "Pump COMM Port"=w569) -> ()  [unwired: 7 in, 2 out]
                                }
                                }
                              }
                              frame #3 {
                                # "Bay 4"
                                n426 = Index Array(array=w581, index=9) -> (element=w578:dbl)
                                n427 = Index Array(array=w581, index=4) -> (element=w579:dbl)
                                n428 = script code="MATLAB script"("P5"=w579, "T4_SP"=w578) -> ()  [unwired: 1 in, 1 out]
                                n429 = Not Equal To 0?(x=w579) -> (x != 0?=w577:bool)
                                n430 = local read "Bay 4"() -> (w584:u16)
                                n431 = Equal?(x=w584, y=1) -> (x = y?=w574:bool)
                                n432 = And(x=w577, y=w573) -> (x .and. y?=w576:bool)
                                n433 = And(x=w574, y=w573) -> (x .and. y?=w575:bool)
                                n434 = case shown="True" w576 {
                                tunnel: w583 -> [w587 w589]
                                tunnel: w579 -> [_ w588]
                                frame False {
                                n435 = call "PumpStop.vi"("Pump Address"="f", "Pump COMM Port"=w587) -> ()  [unwired: 9 in, 1 out]
                                }
                                frame True {
                                n436 = call "PumpDispense.vi"("Flowrate(ul/min)"=w588, "Pump Address"="f", "Pump COMM Port"=w589) -> ()  [unwired: 7 in, 2 out]
                                }
                                }
                                n437 = case shown="True" w575 {
                                tunnel: w578 -> [_ w592]
                                frame False {
                                n438 = local write "Temperature Control 4"(FALSE ("Temperature Control 4")) -> ()
                                }
                                frame True {
                                n439 = local write "Temperature SP 4"(w592) -> ()
                                n440 = local write "Temperature Control 4"(TRUE ("Temperature Control 5")) -> ()
                                }
                                }
                              }
                              frame #4 {
                                # "Bay 5"
                                n441 = Index Array(array=w601, index=5) -> (element=w599:dbl)
                                n442 = Index Array(array=w601, index=4) -> (element=w600:dbl)
                                n443 = script code="MATLAB script"("T5_SP"=w600, "P6"=w599) -> ()  [unwired: 1 in, 1 out]
                                n444 = Not Equal To 0?(x=w599) -> (x != 0?=w596:bool)
                                n445 = And(x=w596, y=w594) -> (x .and. y?=w595:bool)
                                n446 = local read "Bay 5"() -> (w605:u16)
                                n447 = Equal?(x=w605, y=u16 1) -> (x = y?=w597:bool)
                                n448 = And(x=w597, y=w594) -> (x .and. y?=w598:bool)
                                n449 = case shown="True" w598 {
                                tunnel: w600 -> [_ w613]
                                frame False {
                                n450 = local write "Temperature Control 5"(FALSE ("Temperature Control 5")) -> ()
                                }
                                frame True {
                                n451 = local write "Temperature SP 5"(w613) -> ()
                                n452 = local write "Temperature Control 5"(TRUE ("Temperature Control 5")) -> ()
                                }
                                }
                                n453 = case shown="True" w595 {
                                tunnel: w606 -> [w608 w611]
                                tunnel: w599 -> [_ w609]
                                frame False {
                                n454 = call "PumpStop.vi"("Pump Address"="h", "Pump COMM Port"=w608) -> ()  [unwired: 9 in, 1 out]
                                }
                                frame True {
                                n455 = call "PumpDispense.vi"("Flowrate(ul/min)"=w609, "Pump Address"="h", "Pump COMM Port"=w611) -> ()  [unwired: 7 in, 2 out]
                                }
                                }
                              }
                            }
                          }
                          frame #1 {
                            # "Wait till Steady State temperature readings on all bays"
                            n456 = while {
                              tunnel: w616 -> [w617]
                              stop <- w618 stop-if-true
                              n457 = flat-sequence {
                                tunnel: [w621] -> w618
                                tunnel: w617 -> [w620]
                                frame #0 {
                                n458 = Wait (ms)(milliseconds to wait=u32 1500) -> ()  [unwired: 1 out]
                                }
                                frame #1 {
                                n459 = local read "Temp SS? 2"() -> (w624:bool)
                                n460 = local read "Temp SS? 3"() -> (w625:bool)
                                n461 = local read "Temp SS? 4"() -> (w626:bool)
                                n462 = local read "Temp SS? 5"() -> (w627:bool)
                                n463 = local read "Temp SS? 1"() -> (w623:bool)
                                n464 = Not(x=w620) -> (.not. x?=w633:bool)
                                n465 = local read "Stop"() -> (w622:bool)
                                n466 = And(x=w625, y=w626) -> (x .and. y?=w629:bool)
                                n467 = And(x=w623, y=w624) -> (x .and. y?=w630:bool)
                                n468 = And(x=w630, y=w629) -> (x .and. y?=w628:bool)
                                n469 = And(x=w628, y=w627) -> (x .and. y?=w631:bool)
                                n470 = Or(x=w633, y=w631) -> (x .or. y?=w632:bool)
                                n471 = Or(x=w632, y=w622) -> (x .or. y?=w621:bool)
                                }
                              }
                            }
                            n472 = local write "Calculate condition"(TRUE ("Calculate condition")) -> ()
                          }
                          frame #2 {
                            n473 = flat-sequence {
                              tunnel: w636 -> [w638]
                              tunnel: [w638] -> w635
                              tunnel: w635 -> [w642]
                              tunnel: [w642] -> w634
                              frame #0 {
                                n474 = local write "Equlibrating Temperature"(TRUE) -> ()
                              }
                              frame #1 {
                                # "Wait 1.5 system volumes"
                                n475 = local read "tau 2"() -> (w647:dbl)
                                n476 = local read "tau 4"() -> (w651:dbl)
                                n477 = local read "tau 3"() -> (w648:dbl)
                                n478 = local read "tau 5"() -> (w653:dbl)
                                n479 = local read "tau 1"() -> (w646:dbl)
                                n480 = Add(x=w646, y=w647) -> (x+y=w649:dbl)
                                n481 = Add(x=w649, y=w648) -> (x+y=w650:dbl)
                                n482 = Add(x=w650, y=w651) -> (x+y=w652:dbl)
                                n483 = Add(x=w652, y=w653) -> (x+y=w641:dbl)
                                n484 = Multiply(x=w641, y=2.0) -> (x*y=w639:dbl)
                                "Total System Resisdence Time(min)" <- w639
                                n485 = Multiply(x=w639, y=3) -> (x*y=w645:dbl)
                                "total_flush_time" <- w645
                                n486 = Multiply(x=60.0, y=w645) -> (x*y=w644:dbl)
                                n487 = property on="System Flush Wait Time" class="Slide (strict)"("Scale.Maximum"=w644) -> ()  [unwired: 2 in, 2 out]
                                n488 = script code="start = tic;"("total_wait_time"=w644) -> ("??"=w643:errorcluster)  [unwired: 1 in]
                                n489 = while {
                                tunnel: w642 -> [w657]
                                tunnel: w643 -> [w661]
                                stop <- w662 stop-if-true
                                # "Check if system is flushed every 10 seconds"
                                n490 = script code="end1 = toc(start);\nflush_time = 0;\nif end1 > total_wait_time\n   flush_time = 1;\nend\ncurr_wait_time = end1 /60;"("??"=w661) -> ("flush_time"=w665:dbl, "curr_wait_time"=w660:dbl)  [unwired: 1 out]
                                "curr_wait_time" <- w660
                                n491 = Not Equal To 0?(x=w665) -> (x != 0?=w664:bool)
                                n492 = Multiply(x=60.0, y=w660) -> (x*y=w659:dbl)
                                n493 = local read "Stop"() -> (w667:bool)
                                n494 = local write "System Flush Wait Time"(w659) -> ()
                                n495 = Or(x=w664, y=w667) -> (x .or. y?=w663:bool)
                                n496 = Not(x=w657) -> (.not. x?=w656:bool)
                                n497 = Wait (ms)(milliseconds to wait=u32 10000) -> ()  [unwired: 1 out]
                                n498 = Or(x=w663, y=w656) -> (x .or. y?=w662:bool)
                                }
                              }
                            }
                          }
                          frame #3 {
                            # "Collect HPLC Data"
                            n499 = local write "Flushing System"(TRUE ("Flushing System")) -> ()
                            n500 = flat-sequence {
                              tunnel: w670 -> [w677]
                              tunnel: w669 -> [w678]
                              tunnel: w668 -> [w676]
                              frame #0 {
                                n501 = local read "pause for ms"() -> (w673:bool)
                                n502 = case shown="True" w673 {
                                frame False {
                                }
                                frame True {
                                n503 = One Button Dialog(message="Press OK to Analyze Data", button name ("OK")="OK" ("Left Button Text (\"Yes\")")) -> ()  [unwired: 1 out]
                                }
                                }
                              }
                              frame #1 {
                                n504 = flat-sequence {
                                tunnel: [w680] -> w679
                                tunnel: w679 -> [w686]
                                tunnel: w678 -> [w694]
                                tunnel: w677 -> [w696]
                                tunnel: w676 -> [w695]
                                frame #0 {
                                n505 = disable-structure shown="Enabled" {
                                disable-tunnel: [w681 _] -> w680
                                frame Disabled {
                                n506 = local read "COMM Port :: Milligat Pumps"() -> (w682:refnum<visa-resource-name>)
                                n507 = local read "P_tot"() -> (w685:dbl)
                                n508 = Multiply(x=w685, y=2.0) -> (x*y=w681:dbl)
                                n509 = call "PumpDispense.vi"("Flowrate(ul/min)"=w681, "Pump Address"="f", "Pump COMM Port"=w682) -> ()  [unwired: 7 in, 2 out]
                                }
                                frame Enabled {
                                }
                                }
                                }
                                frame #1 {
                                n510 = disable-structure shown="Enabled" {
                                disable-tunnel: w686 -> [w688 _]
                                frame Disabled {
                                n511 = local read "Stop"() -> (w687:bool)
                                n512 = case shown="False" w687 {
                                tunnel: w688 -> [w689 _]
                                frame False {
                                n513 = Divide(x=400.0 ("y"), y=w689) -> (x/y=w691:dbl)
                                n514 = Multiply(x=60000.0, y=w691) -> (x*y=w693:dbl)
                                n515 = Wait (ms)(milliseconds to wait=w693) -> ()  [unwired: 1 out]
                                }
                                frame True {
                                }
                                }
                                }
                                frame Enabled {
                                }
                                }
                                }
                                frame #2 {
                                n516 = while {
                                tunnel: w694 -> [w708]
                                tunnel: w696 -> [w700]
                                tunnel: w695 -> [w702]
                                tunnel: w694 -> [w699]
                                stop <- w703 stop-if-true
                                n517 = flat-sequence {
                                tunnel: w700 -> [_]
                                tunnel: w700 -> [_]
                                tunnel: w699 -> [w709]
                                tunnel: w700 -> [w784]
                                tunnel: w708 -> [_]
                                tunnel: [w803] -> w698
                                tunnel: [w802] -> w697
                                tunnel: w698 -> [w825]
                                tunnel: w697 -> [w824]
                                tunnel: [w844] -> w701
                                tunnel: [w850] -> w706
                                tunnel: w701 -> [w850]
                                tunnel: w700 -> [w849]
                                frame #0 {
                                n518 = local read "COMM Port :: Milligat Pumps"() -> (w711:refnum<visa-resource-name>)
                                n519 = stacked-sequence {
                                tunnel: w711 -> [w714 w726 w744 w749 w758 w771]
                                tunnel: w709 -> [w713 w722 w741 w751 w760 w767]
                                tunnel: 1.0 ("Flowrate(ul/min)") -> [w712 w721 w739 w748 w757 w766]
                                frame #0 {
                                n520 = Index Array(array=w713, index=0) -> (element=w716:dbl)
                                n521 = Greater Than 0?(x=w716) -> (x > 0?=w715:bool)
                                n522 = case shown="True" w715 {
                                tunnel: w714 -> [_ w720]
                                tunnel: w712 -> [_ w718]
                                frame False {
                                }
                                frame True {
                                n523 = call "PumpDispense.vi"("Flowrate(ul/min)"=w718, "Pump Address"="g", "Pump COMM Port"=w720) -> ()  [unwired: 7 in, 2 out]
                                }
                                }
                                }
                                frame #1 {
                                n524 = Index Array(array=w722, index=1) -> (element=w724:dbl)
                                n525 = Greater Than 0?(x=w724) -> (x > 0?=w723:bool)
                                n526 = case shown="True" w723 {
                                tunnel: w721 -> [_ w728]
                                tunnel: w726 -> [_ w727]
                                frame False {
                                }
                                frame True {
                                n527 = local read "Syringe_pump?"() -> (w729:bool)
                                n528 = case shown="True" w729 {
                                tunnel: w728 -> [w731 w736]
                                tunnel: w727 -> [w730 _]
                                frame False {
                                n529 = call "PumpDispense.vi"("Flowrate(ul/min)"=w731, "Pump Address"="j", "Pump COMM Port"=w730) -> ()  [unwired: 7 in, 2 out]
                                }
                                frame True {
                                w733 = u16 0 items=["Infuse", "Withdraw"] ("Run Direction (0:Infuse)")
                                w735 = u32 4 items=["milliliters per hour (ml/hr)", "milliliters per minute (ml/min)", "milliliters per second (ml/sec)", "microliters per hour (ul/hr)", "microliters per minute (ul/min)", "microliters per second (ul/sec)", "nanoliters per hour (nl/hr)", "nanoliters per minute (nl/min)", "nanoliters per second (nl/sec)", "picoliters per hour (pl/hr)", "picoliters per minute (pl/min)", "picoliters per second (pl/sec)"] ("Flow Rate Units (1:ml/min)")
                                w737 = u16 0 items=["Infuse", "Withdraw"] ("Pump Direction (0:Infuse)")
                                (unwired) i8 2 ("Pump Address")
                                n530 = local read "COMM Port:: Harvard Syringe Pump"() -> (w738:refnum<visa-resource-name>)
                                n531 = call <instrlib>:"Configure Flow Rate & Direction.vi"("VISA resource name"=w738, "Pump Direction (0:Infuse)"=w737, "Flow Rate (5.00)"=w736, "Flow Rate Units (1:ml/min)"=w735) -> ("VISA resource name out"=w734:refnum<visa-resource-name>)  [unwired: 10 in, 1 out]
                                n532 = call <instrlib>:"Start Pump.vi"("Run Direction (0:Infuse)"=w733, "VISA resource name"=w734) -> ()  [unwired: 8 in, 2 out]
                                }
                                }
                                }
                                }
                                }
                                frame #2 {
                                n533 = Index Array(array=w741, index=2) -> (element=w742:dbl)
                                n534 = Greater Than 0?(x=w742) -> (x > 0?=w740:bool)
                                n535 = case shown="True" w740 {
                                tunnel: w744 -> [_ w747]
                                tunnel: w739 -> [_ w745]
                                frame False {
                                }
                                frame True {
                                n536 = call "PumpDispense.vi"("Flowrate(ul/min)"=w745, "Pump Address"="i", "Pump COMM Port"=w747) -> ()  [unwired: 7 in, 2 out]
                                }
                                }
                                }
                                frame #3 {
                                n537 = Index Array(array=w751, index=3) -> (element=w752:dbl)
                                n538 = Greater Than 0?(x=w752) -> (x > 0?=w750:bool)
                                n539 = case shown="True" w750 {
                                tunnel: w749 -> [_ w756]
                                tunnel: w748 -> [_ w754]
                                frame False {
                                }
                                frame True {
                                n540 = call "PumpDispense.vi"("Flowrate(ul/min)"=w754, "Pump Address"="e", "Pump COMM Port"=w756) -> ()  [unwired: 7 in, 2 out]
                                }
                                }
                                }
                                frame #4 {
                                n541 = Index Array(array=w760, index=4) -> (element=w761:dbl)
                                n542 = Greater Than 0?(x=w761) -> (x > 0?=w759:bool)
                                n543 = case shown="True" w759 {
                                tunnel: w758 -> [_ w765]
                                tunnel: w757 -> [_ w763]
                                frame False {
                                }
                                frame True {
                                n544 = call "PumpDispense.vi"("Flowrate(ul/min)"=w763, "Pump Address"="f", "Pump COMM Port"=w765) -> ()  [unwired: 7 in, 2 out]
                                }
                                }
                                }
                                frame #5 {
                                n545 = Index Array(array=w767, index=5) -> (element=w769:dbl)
                                n546 = Greater Than 0?(x=w769) -> (x > 0?=w768:bool)
                                n547 = case shown="True" w768 {
                                tunnel: w771 -> [_ w774]
                                tunnel: w766 -> [_ w772]
                                frame False {
                                }
                                frame True {
                                n548 = call "PumpDispense.vi"("Flowrate(ul/min)"=w772, "Pump Address"="h", "Pump COMM Port"=w774) -> ()  [unwired: 7 in, 2 out]
                                }
                                }
                                }
                                }
                                }
                                frame #1 {
                                n549 = while {
                                stop <- w780 stop-if-true
                                n550 = local read "Phase_Sensor_voltage"() -> (w775:dbl)
                                n551 = script code="organic_phase = 0;\nif start_phase_time \n   start_phase_timer = tic;\n   start_phase_time = 0;\nelse\n  %ignore phase sensor values\n  %if not(phase_sensor_val >2.9 && phase_sensor_val <3.8)\n    %    start_phase_timer = tic;\n   %end\n\n   end_phase_time =  toc(start_phase_timer )\n\n   if end_phase_time > 2\n       organic_phase = 1;\n       start_phase_time = 1;\n   end\n\nend"("phase_sensor_val"=w775) -> ("organic_phase"=w777:dbl)  [unwired: 1 in, 1 out]
                                n552 = local read "Stop"() -> (w779:bool)
                                n553 = Not Equal To 0?(x=w777) -> (x != 0?=w778:bool)
                                n554 = Or(x=w778, y=w779) -> (x .or. y?=w780:bool)
                                n555 = Wait (ms)(milliseconds to wait=u32 300) -> ()  [unwired: 1 out]
                                }
                                }
                                frame #2 {
                                n556 = local read "Stop"() -> (w782:bool)
                                n557 = Not(x=w782) -> (.not. x?=w781:bool)
                                n558 = local read "Sample Valve COMM::Port"() -> (w783:refnum<visa-resource-name>)
                                n559 = case shown="True" w781 {
                                tunnel: w784 -> [_ w786]
                                tunnel: w783 -> [_ w785]
                                frame False {
                                }
                                frame True {
                                n560 = flat-sequence {
                                tunnel: w786 -> [w789]
                                tunnel: w785 -> [w798]
                                frame #0 {
                                n561 = local read "Sample Valve COMM::Port"() -> (w792:refnum<visa-resource-name>)
                                n562 = call-poly <vilib>:"Digital Write.vi"("Output Value"=FALSE, "DO Channel"=u8 22, "LINX Resource"=w789) -> ("LINX Resource"=w788:T8)  [unwired: 7 in, 1 out]
                                n563 = flat-sequence {
                                tunnel: w788 -> [w795]
                                tunnel: [w795] -> w787
                                frame #0 {
                                n564 = Wait (ms)(milliseconds to wait=u32 500) -> ()  [unwired: 1 out]
                                }
                                }
                                n565 = call-poly <vilib>:"Digital Write.vi"("Output Value"=TRUE, "DO Channel"=u8 22, "LINX Resource"=w787) -> ()  [unwired: 7 in, 2 out]
                                n566 = call "NanoValve Inject.vi"("VISA resource name"=w792) -> ()  [unwired: 10 in, 1 out]
                                }
                                frame #1 {
                                n567 = Wait (ms)(milliseconds to wait=u32 2000) -> ()  [unwired: 1 out]
                                }
                                frame #2 {
                                n568 = call "NanoValve Load.vi"("VISA resource name"=w798) -> ()  [unwired: 10 in, 1 out]
                                }
                                }
                                }
                                }
                                }
                                frame #3 {
                                n569 = disable-structure shown="Disabled" {
                                frame Disabled {
                                n570 = local read "COMM Port :: Milligat Pumps"() -> (w799:refnum<visa-resource-name>)
                                n571 = call "PumpDispense.vi"("Flowrate(ul/min)"=10.0, "Pump Address"="f", "Pump COMM Port"=w799) -> ()  [unwired: 7 in, 2 out]
                                }
                                frame Enabled {
                                }
                                }
                                }
                                frame #4 {
                                n572 = local read "Stop"() -> (w806:bool)
                                n573 = local read "Bay Parameters"() -> (w802:T3)
                                n574 = Unbundle By Name(w802) -> ("Hplc Wait time(min)"=w804:dbl)
                                n575 = Not(x=w806) -> (.not. x?=w805:bool)
                                n576 = case shown="True" w805 {
                                tunnel: w804 -> [_ w810]
                                tunnel: [errorcluster {"status"=FALSE, "code"=0, "source"=""} ("error out") w809] -> w803
                                tunnel: w802 -> [_ w808]
                                frame False {
                                }
                                frame True {
                                n577 = flat-sequence {
                                tunnel: w810 -> [w812]
                                tunnel: [w822] -> w809
                                tunnel: w808 -> [w821]
                                frame #0 {
                                # "Wait till for HPLC Method"
                                n578 = script code="start = tic;"() -> ("??"=w811:errorcluster)  [unwired: 1 in]
                                n579 = while {
                                tunnel: w812 -> [w814]
                                tunnel: w811 -> [w813]
                                stop <- w820 stop-if-true
                                n580 = Multiply(x=w814, y=60.0) -> (x*y=w815:dbl)
                                n581 = script code="end1 = toc(start);\nflush_time = 0;\nif end1 > hplc_wait_time\n   flush_time = 1;\nend"("??"=w813, "hplc_wait_time"=w815) -> ("flush_time"=w817:dbl)  [unwired: 1 out]
                                n582 = local read "Stop"() -> (w819:bool)
                                n583 = Not Equal To 0?(x=w817) -> (x != 0?=w818:bool)
                                n584 = Or(x=w818, y=w819) -> (x .or. y?=w820:bool)
                                }
                                }
                                frame #1 {
                                n585 = Unbundle By Name(w821) -> ("hplc File Name"=w823:string)
                                n586 = call "hplc_analyze.vi"("File Path"=w823) -> ("error out"=w822:errorcluster)  [unwired: 10 in]
                                }
                                }
                                }
                                }
                                }
                                frame #5 {
                                n587 = Unbundle By Name(w825) -> ("status"=w826:bool)
                                n588 = case shown="True" w826 {
                                tunnel: w824 -> [_ w827]
                                frame False {
                                }
                                frame True {
                                n589 = while {
                                tunnel: w827 -> [w829]
                                stop <- w828 stop-if-true
                                w834 = "An error occured while trying to read HPLC data. " ("message")
                                n590 = local write "Error Message"(w834) -> ()
                                n591 = call <vilib>:"Three Button Dialog.vi"("Right Button Text (\"Cancel\")"="STOP EXPs" ("F button name (\"Cancel\")"), "Center Button Text (\"No\")"="REDO" ("T button name (\"OK\")"), "Left Button Text (\"Yes\")"="REREAD" ("T button name (\"OK\")"), "message"=w834) -> ("Which Button?"=w830:T15)  [unwired: 7 in]
                                n592 = case shown="\"Right Button\"" w830 {
                                tunnel: w829 -> [_ _ w841 _]
                                tunnel: [TRUE TRUE w840 w843] -> w828
                                frame "Right Button" {
                                w836 = TRUE ("Setup Error")
                                n593 = local write "Setup Error"(w836) -> ()
                                n594 = script code="system_error = 1"() -> ()  [unwired: 1 in, 1 out]
                                n595 = local write "Stop"(w836) -> ()
                                }
                                frame "Center Button" {
                                n596 = script code="redo = true;\nopt_ctr = 1;\nCurrExp = CurrExp + 1;\nncall0 = ncall0 +1;\nif req_ctr == req_tot\n       opt_ctr = 3;\n  else\n     req_ctr = req_ctr +1;\nend"() -> ()  [unwired: 1 in, 1 out]
                                }
                                frame "Left Button" {
                                n597 = Unbundle By Name(w841) -> ("hplc File Name"=w842:string)
                                n598 = call "hplc_analyze.vi"("File Path"=w842) -> ("error out"=w838:errorcluster)  [unwired: 10 in]
                                n599 = Unbundle By Name(w838) -> ("status"=w839:bool)
                                n600 = Not(x=w839) -> (.not. x?=w840:bool)
                                }
                                frame "Window Close" {
                                w843 = TRUE
                                n601 = local write "Setup Error"(w843) -> ()
                                n602 = script code="system_error = 1"() -> ()  [unwired: 1 in, 1 out]
                                n603 = local write "Stop"(w843) -> ()
                                }
                                }
                                }
                                }
                                }
                                }
                                frame #6 {
                                n604 = script code="repeat = 0"() -> ("repeat"=w845:dbl)  [unwired: 1 in, 1 out]
                                n605 = Equal To 0?(x=w845) -> (x = 0?=w844:bool)
                                n606 = case shown="False" w844 {
                                frame False {
                                n607 = local read "COMM Port :: Milligat Pumps"() -> (w846:refnum<visa-resource-name>)
                                n608 = call "PumpDispense.vi"("Flowrate(ul/min)"=30.0, "Pump Address"="f", "Pump COMM Port"=w846) -> ()  [unwired: 7 in, 2 out]
                                }
                                frame True {
                                }
                                }
                                }
                                frame #7 {
                                n609 = disable-structure shown="Disabled" {
                                disable-tunnel: w849 -> [w853 _]
                                frame Disabled {
                                n610 = flat-sequence {
                                tunnel: w852 -> [w858]
                                tunnel: [w858] -> _
                                tunnel: [w858] -> w851
                                frame #0 {
                                n611 = Wait (ms)(milliseconds to wait=u32 500) -> ()  [unwired: 1 out]
                                }
                                }
                                n612 = call-poly <vilib>:"Digital Write.vi"("Output Value"=FALSE, "DO Channel"=u8 22, "LINX Resource"=w853) -> ("LINX Resource"=w852:T8)  [unwired: 7 in, 1 out]
                                n613 = call-poly <vilib>:"Digital Write.vi"("Output Value"=TRUE, "DO Channel"=u8 22, "LINX Resource"=w851) -> ()  [unwired: 7 in, 2 out]
                                }
                                frame Enabled {
                                }
                                }
                                }
                                }
                                n614 = local read "Stop"() -> (w707:bool)
                                n615 = Not(x=w702) -> (.not. x?=w705:bool)
                                n616 = Or(x=w707, y=w706) -> (x .or. y?=w704:bool)
                                n617 = Or(x=w704, y=w705) -> (x .or. y?=w703:bool)
                                }
                                }
                                }
                              }
                              frame #2 {
                                n618 = script code="C_measured =Conc;\nFvalues(end +1,:) = [Conc];"() -> ()  [unwired: 1 in, 1 out]
                                n619 = local write "HPLC Analysis"(TRUE ("HPLC Analysis")) -> ()
                              }
                            }
                            "System Flushed?" <- TRUE ("System Flushed?")
                          }
                          frame #4 {
                            n620 = local read "Stop"() -> (w862:bool)
                            n621 = Not(x=w862) -> (.not. x?=w861:bool)
                            n622 = case shown="True" w861 {
                              tunnel: [1.0 w867] -> w863
                              frame False {
                              }
                              frame True {
                                # "Save data to excel file"
                                n623 = local read "Total Number of Experiments"() -> (w865:dbl)
                                n624 = script code="if not(system_error) && not(redo)\n  if opt_ctr == 1\n        f(req_ctr,:) = [-(C_measured) sqrt(eps)];  \n     %f(req_ctr,:) = [-C_measured/total_wait_time sqrt(eps)];  \n  end\n  temp_write = [CurrExp, f(req_ctr,1), C_measured];\n  lastrowStr4 = num2str(lastrow4);\n  xlSheets.Item(idx4).Range(strcat('A',lastrowStr4,':',lastcol4,lastrowStr4)).Value2 =  temp_write;\n  lastrow4 = lastrow4 +1;\n  xlWorkbook.SaveAs(xl_file);\n  allHPLCData(end+1,:) =  [CurrExp new_x(:)' f(req_ctr,1) C_measured]\n  %allHPLCFile(end+1,:) = [num2str(CurrExp) hplc_file];\n\n  opt_ctr = 1;\n  CurrExp = CurrExp + 1;\n  terminate = 0;\n\n    if is_first_set_of_exp\n       ncall0 = size(f,1);\n       is_first_set_of_exp = false;\n    else\n       ncall0 = ncall0 +1;% size(f,1); % update function call counter\n    end\n    [fbestn,jbest] = min(f(:,1)); % best function value\n\n    if fbestn < fbest\n        fbest = fbestn;\n        xbest = x(jbest,:);\n        ncall0,xbest,fbest % display current number of function values,\n        % best point and function value if fbest has changed\n        nstop0 = 0;\n   \n    end\n  \n      % check stopping criterion\n    if nstop0 >= nstop  || ncall0 >= ncall\n       terminate = 1;\n       lastrowStr_temp = num2str(10);\n       lastcol_temp =  xlcolumnletter(length(xbest)+1);\n       xlSheets.Item(idx3).Range(strcat('B',lastrowStr_temp,':',lastcol_temp,lastrowStr_temp)).Value2 =  xbest;\n       xlWorkbook.SaveAs(xl_file);\n    end\n\n    if req_ctr == req_tot\n        if ncall >= minfcall && fbestn > fbest\n           nstop0 = nstop0 + 1;\n        end\n       opt_ctr = 3;\n    else\n       req_ctr = req_ctr +1;\n    end\n\n   save(matlabsavefile);\nend"("ncall"=w865) -> ("terminate"=w867:dbl, "ncall0"=w866:dbl)  [unwired: 1 in, 1 out]
                                n625 = local write "Current Experiment"(w866) -> ()
                              }
                            }
                          }
                          frame #5 {
                            n626 = local read "Num_exp_till_pause"() -> (w869:i32)
                            n627 = Increment(x=w869) -> (x+1=w868:i32)
                            n628 = local write "Num_exp_till_pause"(w868) -> ()
                          }
                          frame #6 {
                            # "Pause System"
                            n629 = local read "Bay Parameters"() -> (w877:T3)
                            n630 = Unbundle By Name(w877) -> ("Num_conditons_per_wait"=w876:dbl)
                            n631 = local read "Num_exp_till_pause"() -> (w875:i32)
                            n632 = Equal?(x=w876, y=w875) -> (x = y?=w874:bool)
                            n633 = local read "Run_Stop_cluster"() -> (w871:T5)
                            n634 = Unbundle By Name(w871) -> ("Stop Run Button"=w873:bool)
                            n635 = Or(x=w873, y=w874) -> (x .or. y?=w872:bool)
                            n636 = case shown="True" w872 {
                              tunnel: w876 -> [w880 _]
                              tunnel: w875 -> [w881 _]
                              tunnel: w871 -> [_ w883]
                              frame False {
                                n637 = Greater?(x=w881, y=w880) -> (0:w879:bool)
                                n638 = case shown="True" w879 {
                                frame False {
                                }
                                frame True {
                                n639 = local write "Num_exp_till_pause"(0 ("Num_exp_till_pause")) -> ()
                                }
                                }
                              }
                              frame True {
                                n640 = flat-sequence {
                                tunnel: w883 -> [w911]
                                frame #0 {
                                w887 = string[] ["e", "f", "g", "h", "i", "j"]
                                # "Turn off pumps and stop controling temperature"
                                n641 = stacked-sequence {
                                frame #0 {
                                n642 = local write "Temperature Control 1"(FALSE ("Temperature Control 1")) -> ()
                                }
                                frame #1 {
                                n643 = local write "Temperature Control 2"(FALSE ("Temperature Control 2")) -> ()
                                }
                                frame #2 {
                                n644 = local write "Temperature Control 3"(FALSE ("Temperature Control 3")) -> ()
                                }
                                frame #3 {
                                n645 = local write "Temperature Control 4"(FALSE ("Temperature Control 4")) -> ()
                                }
                                frame #4 {
                                n646 = local write "Temperature Control 5"(FALSE ("Temperature Control 5")) -> ()
                                }
                                }
                                n647 = local read "COMM Port:: Harvard Syringe Pump"() -> (w885:refnum<visa-resource-name>)
                                n648 = local read "Syringe_pump?"() -> (w884:bool)
                                n649 = local read "COMM Port :: Milligat Pumps"() -> (w886:refnum<visa-resource-name>)
                                n650 = Array Size(array=w887) -> (size(s)=w888:i32)
                                n651 = case shown="True" w884 {
                                tunnel: w885 -> [_ w896]
                                frame False {
                                }
                                frame True {
                                n652 = call <instrlib>:"Stop Pump.vi"("VISA resource name"=w896) -> ()  [unwired: 9 in, 2 out]
                                }
                                }
                                n653 = for {
                                N: w888 -> [_]
                                tunnel: w887 -> [w895] mode=indexing
                                tunnel: w886 -> [w894]
                                n654 = call "PumpStop.vi"("Pump Address"=w895, "Pump COMM Port"=w894) -> ()  [unwired: 9 in, 1 out]
                                }
                                }
                                frame #1 {
                                n655 = local read "Stop"() -> (w899:bool)
                                n656 = Not(x=w899) -> (.not. x?=w898:bool)
                                n657 = case shown="True" w898 {
                                frame False {
                                }
                                frame True {
                                n658 = while {
                                stop <- w905 stop-if-true
                                # "Wait till user confirms system resume"
                                n659 = Two Button Dialog(message="System is currently paused. Refill Syringes, flush lines, then press OK to continue optimization.\nOr Redo to repeat condition ", 1:"REDO" ("F button name (\"Cancel\")"), 2:"OK" ("Left Button Text (\"Yes\")")) -> (T button?=w901:bool)
                                n660 = case shown="False" w901 {
                                tunnel: [TRUE TRUE] -> w900
                                frame False {
                                n661 = script code="redo = true;"() -> ()  [unwired: 1 in, 1 out]
                                }
                                frame True {
                                }
                                }
                                n662 = local read "Stop"() -> (w906:bool)
                                n663 = Or(x=w900, y=w906) -> (x .or. y?=w905:bool)
                                }
                                }
                                }
                                n664 = local write "stop_xl_write"(TRUE ("stop_xl_write")) -> ()
                                }
                                frame #2 {
                                n665 = local write "Num_exp_till_pause"(0 ("Num_exp_till_pause")) -> ()
                                n666 = Bundle By Name(cluster=w911, "Stop Run Button"=FALSE) -> (w909:T5)
                                n667 = local write "Run_Stop_cluster"(w909) -> ()
                                }
                                }
                              }
                            }
                          }
                          frame #7 {
                            w914 = FALSE
                            n668 = local write "Equlibrating Temperature"(w914) -> ()
                            n669 = local write "Calculate condition"(w914) -> ()
                            n670 = local write "Flushing System"(w914) -> ()
                            n671 = local write "HPLC Analysis"(w914) -> ()
                            n672 = local write "stop_xl_write"(TRUE ("stop_xl_write")) -> ()
                          }
                        }
                        n673 = while {
                          stop <- w972 stop-if-true
                          n674 = flat-sequence {
                            frame #0 {
                              n675 = script code="temp_time_cond= [CurrExp, 1, P1, P2, P3, P4, P5,P6, T1, T2, T3, T4, T5, T1_SP, T2_SP, T3_SP, T4_SP, T5_SP, F1, F2, Pres1, Pres2];\n   lastrowStr1 = num2str(lastrow1);\n   xlSheets.Item(idx1).Range(strcat('A',lastrowStr1,':',lastcol1,lastrowStr1)).Value2 =   temp_time_cond;\n   lastrow1 = lastrow1+1;\n  xlWorkbook.SaveAs(xl_file);"() -> ()  [unwired: 1 in, 1 out]
                            }
                            frame #1 {
                              n676 = Wait (ms)(milliseconds to wait=u32 30000) -> ()  [unwired: 1 out]
                            }
                          }
                          n677 = local read "Stop"() -> (w973:bool)
                          n678 = local read "stop_xl_write"() -> (w971:bool)
                          n679 = Or(x=w971, y=w973) -> (x .or. y?=w972:bool)
                        }
                      }
                    }
                  }
                  frame True {
                    # "STANDBY MODE"
                    n680 = Add(x=w976, y=2.0) -> (x+y=w978:dbl)
                  }
                }
                n681 = Greater?(x=w434, y=w435) -> (0:w443:bool)
                n682 = Equal?(x=w441, y=1.0) -> (x = y?=w436:bool)
                n683 = local read "Stop"() -> (w444:bool)
                n684 = Or(x=w444, y=w443) -> (x .or. y?=w440:bool)
                n685 = Or(x=w436, y=w440) -> (x .or. y?=w439:bool)
                n686 = case shown="True" w436 {
                  frame False {
                  }
                  frame True {
                    n687 = local write "Stop"(TRUE ("Stop")) -> ()
                  }
                }
                "Optimization_loop_index" <- w445
              }
            }
          }
          n688 = while {
            tunnel: w424 -> [w1081]
            stop <- w1082 stop-if-true
            n689 = local read "Temperature Control 3"() -> (w1077:bool)
            n690 = local read "Debug_run_button"() -> (w1078:bool)
            n691 = Not(x=w1078) -> (.not. x?=w1080:bool)
            n692 = And(x=w1080, y=w1077) -> (x .and. y?=w1079:bool)
            n693 = case shown="True" w1079 {
              tunnel: w1081 -> [_ w1111]
              frame False {
                n694 = local write "Temp SS? 3"(TRUE) -> ()
              }
              frame True {
                # "Bay 3 Temperature Controller"
                n695 = local read "Temperature SP 3"() -> (w1085:dbl)
                n696 = local read "Temperature 3"() -> (w1088:dbl)
                n697 = Subtract(x=w1088, y=w1085) -> (x-y=w1097:dbl)
                n698 = Absolute Value(x=w1097) -> (abs(x)=w1099:dbl)
                n699 = Less Or Equal?(x=w1099, y=1.2) -> (x <= y?=w1096:bool)
                n700 = local write "Temp SS? 3"(w1096) -> ()
                n701 = local read "SSR Duration 3"() -> (w1106:dbl)
                n702 = call-poly <vilib>:"PID Online Autotuning.vi"("setpoint"=w1085, "manipulated variable"=w1106, "autotuning parameters"=T7 {"type of controller"=enum."PID", "relay cycles"=3, "relay amplitude"=1.0, "control specifications"=enum."Normal", "PV noise level"=0.1} ("Autotuning Parameters R1"), "process variable"=w1088, "PID gains in"=T6 {"Proportional gain Kc"=0.38538, "Integral time Ti (sec)"=0.524375, "Derivative time Ti (sec)"=0.12585} ("PID gains 2")) -> ("setpoint out"=w1104:dbl, "process variable out"=w1105:dbl, "PID gains out"=w1108:T14)  [unwired: 6 in, 2 out]
                n703 = Greater?(x=w1085, y=w1088) -> (0:w1095:bool)
                n704 = call <vilib>:"PID Autotuning (Temperature).vi"("desired temperature"=w1104, "measured temperature"=w1105, "PID gains in"=w1108, "output range"=cluster{"output high":dbl, "output low":dbl} {"output high"=3.0, "output low"=-1.0} ("Output range")) -> ("output"=w1101:dbl)  [unwired: 12 in, 3 out]
                n705 = Multiply(x=1000.0, y=w1101) -> (x*y=w1103:dbl)
                n706 = local write "SSR Duration 3"(w1101) -> ()
                n707 = Greater Than 0?(x=w1103) -> (x > 0?=w1094:bool)
                n708 = And(x=w1094, y=w1095) -> (x .and. y?=w1092:bool)
                n709 = Subtract(x=w1088, y=10.0) -> (x-y=w1090:dbl)
                n710 = Less?(x=w1090, y=w1085) -> (x < y?=w1093:bool)
                n711 = And(x=w1093, y=w1092) -> (x .and. y?=w1091:bool)
                n712 = case shown="True" w1091 {
                  tunnel: [errorcluster {"status"=FALSE, "code"=0, "source"=""} ("error out") w1124] -> _
                  tunnel: 4 -> [_ w1125]
                  tunnel: [w1116 w1123] -> _
                  tunnel: w1111 -> [w1116 w1122]
                  tunnel: w1103 -> [w1115 w1121]
                  tunnel: [0.0 w1120] -> w1086
                  tunnel: w1085 -> [_ w1119]
                  frame False {
                    n713 = Absolute Value(x=w1115) -> (abs(x)=w1117:dbl)
                    n714 = Wait (ms)(milliseconds to wait=w1117) -> ()  [unwired: 1 out]
                  }
                  frame True {
                    n715 = call "TurnOnRelayArduino.vi"("channel"=w1125, "duration"=w1121, "LINX Resource"=w1122) -> ("error out"=w1124:errorcluster, "LINX Resource Out"=w1123:T8)  [unwired: 7 in]
                    n716 = script code="tempdiff3= SP3 - T3;\nif tempdiff3 > 10\n  if slope3 < .01\n     temp_check3 = temp_check3 + 1;\n  else\n      temp_check3 =0;\n  end\nend\n\nif temp_check3 > 9\n  temp_error3 = 1\nend"("SP3"=w1119) -> ("temp_error3"=w1120:dbl)  [unwired: 1 in, 1 out]
                  }
                }
                n717 = Not Equal To 0?(x=w1086) -> (x != 0?=w1087:bool)
                n718 = case shown="True" w1087 {
                  frame False {
                  }
                  frame True {
                    n719 = local write "Error Message"("Bay 3 Temperature Heating Error") -> ()
                  }
                }
                n720 = case shown="True" w1087 {
                  tunnel: w1087 -> [_ w1113]
                  frame False {
                  }
                  frame True {
                    n721 = local write "Stop"(w1113) -> ()
                  }
                }
              }
            }
            n722 = Wait (ms)(milliseconds to wait=u32 400) -> ()  [unwired: 1 out]
            n723 = local read "Stop"() -> (w1082:bool)
          }
          n724 = while {
            tunnel: w424 -> [w1033]
            stop <- w1032 stop-if-true
            n725 = local read "Debug_run_button"() -> (w1028:bool)
            n726 = Not(x=w1028) -> (.not. x?=w1031:bool)
            n727 = Wait (ms)(milliseconds to wait=u32 400) -> ()  [unwired: 1 out]
            n728 = local read "Temperature Control 4"() -> (w1030:bool)
            n729 = And(x=w1031, y=w1030) -> (x .and. y?=w1029:bool)
            n730 = case shown="True" w1029 {
              tunnel: w1033 -> [_ w1061]
              frame False {
                n731 = local write "Temp SS? 4"(TRUE ("Temp SS? 4")) -> ()
              }
              frame True {
                # "Bay 4 Temperature Controller"
                n732 = local read "Temperature SP 4"() -> (w1038:dbl)
                n733 = local read "Temperature 4"() -> (w1041:dbl)
                n734 = Subtract(x=w1041, y=w1038) -> (x-y=w1048:dbl)
                n735 = Absolute Value(x=w1048) -> (abs(x)=w1050:dbl)
                n736 = Less Or Equal?(x=w1050, y=1.2) -> (x <= y?=w1047:bool)
                n737 = local write "Temp SS? 4"(w1047) -> ()
                n738 = local read "SSR Duration 4"() -> (w1051:dbl)
                n739 = call-poly <vilib>:"PID Online Autotuning.vi"("setpoint"=w1038, "manipulated variable"=w1051, "autotuning parameters"=T7 {"type of controller"=enum."PID", "relay cycles"=3, "relay amplitude"=1.0, "control specifications"=enum."Normal", "PV noise level"=0.1} ("Autotuning Parameters R1"), "process variable"=w1041, "PID gains in"=T6 {"Proportional gain Kc"=0.38538, "Integral time Ti (sec)"=0.524375, "Derivative time Ti (sec)"=0.12585} ("PID gains 2")) -> ("setpoint out"=w1053:dbl, "process variable out"=w1054:dbl, "PID gains out"=w1056:T14)  [unwired: 6 in, 2 out]
                n740 = call <vilib>:"PID Autotuning (Temperature).vi"("desired temperature"=w1053, "measured temperature"=w1054, "PID gains in"=w1056, "output range"=cluster{"output high":dbl, "output low":dbl} {"output high"=3.0, "output low"=-1.0} ("Output range")) -> ("output"=w1052:dbl)  [unwired: 12 in, 3 out]
                n741 = Subtract(x=w1041, y=10.0) -> (x-y=w1040:dbl)
                n742 = Less?(x=w1040, y=w1038) -> (x < y?=w1042:bool)
                n743 = Multiply(x=1000.0, y=w1052) -> (x*y=w1060:dbl)
                n744 = Greater?(x=w1038, y=w1041) -> (0:w1046:bool)
                n745 = Greater Than 0?(x=w1060) -> (x > 0?=w1045:bool)
                n746 = local write "SSR Duration 4"(w1052) -> ()
                n747 = And(x=w1045, y=w1046) -> (x .and. y?=w1044:bool)
                n748 = And(x=w1042, y=w1044) -> (x .and. y?=w1043:bool)
                n749 = case shown="True" w1043 {
                  tunnel: [errorcluster {"status"=FALSE, "code"=0, "source"=""} ("error out") w1075] -> _
                  tunnel: 5 -> [_ w1076]
                  tunnel: [w1067 w1074] -> _
                  tunnel: w1061 -> [w1067 w1073]
                  tunnel: w1060 -> [w1066 w1072]
                  tunnel: w1038 -> [_ w1071]
                  tunnel: [0.0 w1070] -> w1037
                  frame False {
                    n750 = Absolute Value(x=w1066) -> (abs(x)=w1068:dbl)
                    n751 = Wait (ms)(milliseconds to wait=w1068) -> ()  [unwired: 1 out]
                  }
                  frame True {
                    n752 = call "TurnOnRelayArduino.vi"("channel"=w1076, "duration"=w1072, "LINX Resource"=w1073) -> ("error out"=w1075:errorcluster, "LINX Resource Out"=w1074:T8)  [unwired: 7 in]
                    n753 = script code="tempdiff4= SP4 - T4;\nif tempdiff4 > 10\n  if slope4 < .01\n     temp_check4 = temp_check4 + 1;\n  else\n      temp_check4 =0;\n  end\nend\n\nif temp_check4 > 9\n  temp_error4 = 1\nend"("SP4"=w1071) -> ("temp_error4"=w1070:dbl)  [unwired: 1 in, 1 out]
                  }
                }
                n754 = Not Equal To 0?(x=w1037) -> (x != 0?=w1036:bool)
                n755 = case shown="True" w1036 {
                  frame False {
                  }
                  frame True {
                    n756 = local write "Error Message"("Bay 4 Temperature Heating Error") -> ()
                  }
                }
                n757 = case shown="True" w1036 {
                  tunnel: w1036 -> [_ w1064]
                  frame False {
                  }
                  frame True {
                    n758 = local write "Stop"(w1064) -> ()
                  }
                }
              }
            }
            n759 = local read "Stop"() -> (w1032:bool)
          }
          n760 = while {
            stop <- w428 stop-if-true
            n761 = script code="TempArr1=circshift(TempArr1,9);\nTempArr2=circshift(TempArr2,9);\nTempArr3=circshift(TempArr3,9);\nTempArr4=circshift(TempArr4,9);\nTempArr5=circshift(TempArr5,9);\n\nTempArr1(10)=T1;\nTempArr2(10)=T2;\nTempArr3(10)=T3;\nTempArr4(10)=T4;\nTempArr5(10)=T5;\n\n[slope1 temp] = polyfit([1,2,3,4,5,6,7,8,9,10]',TempArr1,1);\nslope1 = slope1(1);\n[slope2 temp] = polyfit([1,2,3,4,5,6,7,8,9,10]',TempArr2,1);\nslope2= slope2(1);\n[slope3 temp] = polyfit([1,2,3,4,5,6,7,8,9,10]',TempArr3,1);\nslope3 = slope3(1);\n[slope4 temp] = polyfit([1,2,3,4,5,6,7,8,9,10]',TempArr4,1);\nslope4 = slope4(1);\n[slope5 temp] = polyfit([1,2,3,4,5,6,7,8,9,10]',TempArr5,1);\nslope5 = slope5(1);"() -> ()  [unwired: 1 in, 1 out]
            n762 = Wait (ms)(milliseconds to wait=u32 600) -> ()  [unwired: 1 out]
            n763 = local read "Stop"() -> (w428:bool)
          }
          n764 = while {
            tunnel: w424 -> [w984]
            stop <- w983 stop-if-true
            n765 = local read "Debug_run_button"() -> (w980:bool)
            n766 = Not(x=w980) -> (.not. x?=w982:bool)
            n767 = local read "Temperature Control 5"() -> (w979:bool)
            n768 = And(x=w982, y=w979) -> (x .and. y?=w981:bool)
            n769 = case shown="True" w981 {
              tunnel: w984 -> [_ w1012]
              frame False {
                n770 = local write "Temp SS? 5"(TRUE ("Temp SS? 5")) -> ()
              }
              frame True {
                # "Bay 5 Temperature Controller"
                n771 = local read "SSR Duration 5"() -> (w1002:dbl)
                n772 = local read "Temperature SP 5"() -> (w988:dbl)
                n773 = local read "Temperature 5"() -> (w991:dbl)
                n774 = Subtract(x=w991, y=w988) -> (x-y=w999:dbl)
                n775 = Absolute Value(x=w999) -> (abs(x)=w1001:dbl)
                n776 = Less Or Equal?(x=w1001, y=1.2) -> (x <= y?=w998:bool)
                n777 = local write "Temp SS? 5"(w998) -> ()
                n778 = call-poly <vilib>:"PID Online Autotuning.vi"("setpoint"=w988, "manipulated variable"=w1002, "autotuning parameters"=T7 {"type of controller"=enum."PID", "relay cycles"=3, "relay amplitude"=1.0, "control specifications"=enum."Normal", "PV noise level"=0.1} ("Autotuning Parameters R1"), "process variable"=w991, "PID gains in"=T6 {"Proportional gain Kc"=0.38538, "Integral time Ti (sec)"=0.524375, "Derivative time Ti (sec)"=0.12585} ("PID gains 2")) -> ("setpoint out"=w1004:dbl, "process variable out"=w1005:dbl, "PID gains out"=w1007:T14)  [unwired: 6 in, 2 out]
                n779 = call <vilib>:"PID Autotuning (Temperature).vi"("desired temperature"=w1004, "measured temperature"=w1005, "PID gains in"=w1007, "output range"=cluster{"output high":dbl, "output low":dbl} {"output high"=3.0, "output low"=-1.0} ("Output range")) -> ("output"=w1003:dbl)  [unwired: 12 in, 3 out]
                n780 = Multiply(x=1000.0, y=w1003) -> (x*y=w1011:dbl)
                n781 = Greater?(x=w988, y=w991) -> (0:w996:bool)
                n782 = Greater Than 0?(x=w1011) -> (x > 0?=w997:bool)
                n783 = local write "SSR Duration 5"(w1003) -> ()
                n784 = And(x=w997, y=w996) -> (x .and. y?=w994:bool)
                n785 = Subtract(x=w991, y=10.0) -> (x-y=w992:dbl)
                n786 = Greater?(x=w992, y=w988) -> (0:w995:bool)
                n787 = And(x=w995, y=w994) -> (x .and. y?=w993:bool)
                n788 = case shown="True" w993 {
                  tunnel: [errorcluster {"status"=FALSE, "code"=0, "source"=""} ("error out") w1026] -> _
                  tunnel: 6 -> [_ w1027]
                  tunnel: [w1018 w1025] -> _
                  tunnel: w1012 -> [w1018 w1024]
                  tunnel: w1011 -> [w1017 w1023]
                  tunnel: [0.0 w1022] -> w989
                  tunnel: w988 -> [_ w1021]
                  frame False {
                    n789 = Absolute Value(x=w1017) -> (abs(x)=w1019:dbl)
                    n790 = Wait (ms)(milliseconds to wait=w1019) -> ()  [unwired: 1 out]
                  }
                  frame True {
                    n791 = call "TurnOnRelayArduino.vi"("channel"=w1027, "duration"=w1023, "LINX Resource"=w1024) -> ("error out"=w1026:errorcluster, "LINX Resource Out"=w1025:T8)  [unwired: 7 in]
                    n792 = script code="tempdiff5= SP5 - T5;\n\nif tempdiff5 > 10\n  if slope5 < .01\n     temp_check5 = temp_check5 + 1;\n  else\n      temp_check5 =0;\n  end\nend\n\nif temp_check5 >9\n  temp_error5 = 1\nend"("SP5"=w1021) -> ("temp_error5"=w1022:dbl)  [unwired: 1 in, 1 out]
                  }
                }
                n793 = Not Equal To 0?(x=w989) -> (x != 0?=w987:bool)
                n794 = case shown="True" w987 {
                  frame False {
                  }
                  frame True {
                    n795 = local write "Error Message"("Bay 5 Temperature Heating Error") -> ()
                  }
                }
                n796 = case shown="True" w987 {
                  tunnel: w987 -> [_ w1015]
                  frame False {
                  }
                  frame True {
                    n797 = local write "Stop"(w1015) -> ()
                  }
                }
              }
            }
            n798 = Wait (ms)(milliseconds to wait=u32 400) -> ()  [unwired: 1 out]
            n799 = local read "Stop"() -> (w983:bool)
          }
        }
      }
      n800 = local read "IR Sensor Device"() -> (w55:T2)
      n801 = while {
        shift-right: [w152] -> _
        shift-left: w55 -> [w153]
        tunnel: errorcluster {"status"=FALSE, "code"=0, "source"=""} ("error out") -> [w151]
        stop <- w177 stop-if-true
        w168 = u8 7 items=["RAM IR raw  Ch1"=4, "RAM IR raw  Ch2"=5, "RAM T_A"=6, "RAM T_OBJ1"=7, "RAM T_OBJ2"=8, "EEPROM_To_max"=32, "EEPROM_To_min"=33, "EEPROM_PWM_CTRL"=34, "EEPROM_Ta_range"=35, "EEPROM_Emissivity_CorrCoeff"=36, "EEPROM_SMBus Address"=46, "EEPROM_ConfigReg"=37] ("Melexis_Cmmds")
        w170 = u8 7 items=["RAM IR raw  Ch1"=4, "RAM IR raw  Ch2"=5, "RAM T_A"=6, "RAM T_OBJ1"=7, "RAM T_OBJ2"=8, "EEPROM_To_max"=32, "EEPROM_To_min"=33, "EEPROM_PWM_CTRL"=34, "EEPROM_Ta_range"=35, "EEPROM_Emissivity_CorrCoeff"=36, "EEPROM_SMBus Address"=46, "EEPROM_ConfigReg"=37] ("Melexis_Cmmds")
        w169 = u8 7 items=["RAM IR raw  Ch1"=4, "RAM IR raw  Ch2"=5, "RAM T_A"=6, "RAM T_OBJ1"=7, "RAM T_OBJ2"=8, "EEPROM_To_max"=32, "EEPROM_To_min"=33, "EEPROM_PWM_CTRL"=34, "EEPROM_Ta_range"=35, "EEPROM_Emissivity_CorrCoeff"=36, "EEPROM_SMBus Address"=46, "EEPROM_ConfigReg"=37] ("Melexis_Cmmds")
        w174 = u8 7 items=["RAM IR raw  Ch1"=4, "RAM IR raw  Ch2"=5, "RAM T_A"=6, "RAM T_OBJ1"=7, "RAM T_OBJ2"=8, "EEPROM_To_max"=32, "EEPROM_To_min"=33, "EEPROM_PWM_CTRL"=34, "EEPROM_Ta_range"=35, "EEPROM_Emissivity_CorrCoeff"=36, "EEPROM_SMBus Address"=46, "EEPROM_ConfigReg"=37] ("Melexis_Cmmds")
        w179 = u8 7 items=["RAM IR raw  Ch1"=4, "RAM IR raw  Ch2"=5, "RAM T_A"=6, "RAM T_OBJ1"=7, "RAM T_OBJ2"=8, "EEPROM_To_max"=32, "EEPROM_To_min"=33, "EEPROM_PWM_CTRL"=34, "EEPROM_Ta_range"=35, "EEPROM_Emissivity_CorrCoeff"=36, "EEPROM_SMBus Address"=46, "EEPROM_ConfigReg"=37] ("Melexis_Cmmds")
        # "Bay 5 Temperature Read"
        # "Bay 4 Temperature Read"
        # "Bay 3 Temperature Read"
        # "Bay 2 Temperature Read"
        # "Bay 1 Temperature Read"
        n802 = local read "Stop"() -> (w177:bool)
        n803 = call "IRSensorNIRead.vi"("error in (no error)"=w151, "Melexis_Cmmds"=w179, "Address"=u8 1, "device reference"=w153) -> ("error out"=w150:errorcluster, "Temperature"=w180:dbl, "device reference out"=w176:T2)  [unwired: 5 in]
        n804 = local write "error out"(w150) -> ()
        n805 = Unbundle By Name(w150) -> ("status"=w149:bool)
        n806 = call-poly <vilib>:"PID Control Input Filter.vi"("input"=w180) -> ("output"=w147:dbl)  [unwired: 4 in]
        n807 = case shown="True" w149 {
          tunnel: w147 -> [w189 _]
          tunnel: [w189 w190] -> w148
          frame False {
            n808 = local write "Temperature 1"(w189) -> ()
          }
          frame True {
            n809 = local read "Temperature 1"() -> (w190:dbl)
          }
        }
        n810 = flat-sequence {
          tunnel: w176 -> [w199]
          tunnel: [w199] -> _
          tunnel: [w199] -> w175
          frame #0 {
            n811 = Wait (ms)(milliseconds to wait=u32 100) -> ()  [unwired: 1 out]
          }
        }
        n812 = call "IRSensorNIRead.vi"("error in (no error)"=w151, "Melexis_Cmmds"=w174, "Address"=u8 2, "device reference"=w175) -> ("error out"=w146:errorcluster, "Temperature"=w172:dbl, "device reference out"=w171:T2)  [unwired: 5 in]
        n813 = Unbundle By Name(w146) -> ("status"=w145:bool)
        n814 = local write "error out"(w146) -> ()
        n815 = call-poly <vilib>:"PID Control Input Filter.vi"("input"=w172) -> ("output"=w144:dbl)  [unwired: 4 in]
        n816 = case shown="True" w145 {
          tunnel: w144 -> [w187 _]
          tunnel: [w187 w188] -> w143
          frame False {
            n817 = local write "Temperature 2"(w187) -> ()
          }
          frame True {
            n818 = local read "Temperature 2"() -> (w188:dbl)
          }
        }
        n819 = flat-sequence {
          tunnel: w171 -> [w197]
          tunnel: [w197] -> _
          tunnel: [w197] -> w164
          frame #0 {
            n820 = Wait (ms)(milliseconds to wait=u32 100) -> ()  [unwired: 1 out]
          }
        }
        n821 = call "IRSensorNIRead.vi"("error in (no error)"=w151, "Melexis_Cmmds"=w169, "Address"=u8 3, "device reference"=w164) -> ("error out"=w140:errorcluster, "Temperature"=w159:dbl, "device reference out"=w163:T2)  [unwired: 5 in]
        n822 = local write "error out"(w140) -> ()
        n823 = Unbundle By Name(w140) -> ("status"=w139:bool)
        n824 = call-poly <vilib>:"PID Control Input Filter.vi"("input"=w159) -> ("output"=w142:dbl)  [unwired: 4 in]
        n825 = case shown="False" w139 {
          tunnel: w142 -> [w185 _]
          tunnel: [w185 w186] -> w141
          frame False {
            n826 = local write "Temperature 3"(w185) -> ()
          }
          frame True {
            n827 = local read "Temperature 3"() -> (w186:dbl)
          }
        }
        n828 = flat-sequence {
          tunnel: w163 -> [w195]
          tunnel: [w195] -> w161
          frame #0 {
            n829 = Wait (ms)(milliseconds to wait=u32 100) -> ()  [unwired: 1 out]
          }
        }
        n830 = call "IRSensorNIRead.vi"("error in (no error)"=w151, "Melexis_Cmmds"=w170, "Address"=u8 4, "device reference"=w161) -> ("error out"=w135:errorcluster, "Temperature"=w158:dbl, "device reference out"=w162:T2)  [unwired: 5 in]
        n831 = local write "error out"(w135) -> ()
        n832 = Unbundle By Name(w135) -> ("status"=w136:bool)
        n833 = call-poly <vilib>:"PID Control Input Filter.vi"("input"=w158) -> ("output"=w138:dbl)  [unwired: 4 in]
        n834 = case shown="True" w136 {
          tunnel: w138 -> [w183 _]
          tunnel: [w183 w184] -> w137
          frame False {
            n835 = local write "Temperature 4"(w183) -> ()
          }
          frame True {
            n836 = local read "Temperature 4"() -> (w184:dbl)
          }
        }
        n837 = flat-sequence {
          tunnel: w162 -> [w193]
          tunnel: [w193] -> w160
          frame #0 {
            n838 = Wait (ms)(milliseconds to wait=u32 100) -> ()  [unwired: 1 out]
          }
        }
        n839 = call "IRSensorNIRead.vi"("error in (no error)"=w151, "Melexis_Cmmds"=w168, "Address"=u8 5, "device reference"=w160) -> ("error out"=w131:errorcluster, "Temperature"=w157:dbl, "device reference out"=w156:T2)  [unwired: 5 in]
        n840 = flat-sequence {
          tunnel: w156 -> [w191]
          tunnel: [w191] -> w152
          frame #0 {
            n841 = Wait (ms)(milliseconds to wait=u32 100) -> ()  [unwired: 1 out]
          }
        }
        n842 = call-poly <vilib>:"PID Control Input Filter.vi"("input"=w157) -> ("output"=w134:dbl)  [unwired: 4 in]
        n843 = local write "error out"(w131) -> ()
        n844 = Unbundle By Name(w131) -> ("status"=w132:bool)
        n845 = Build Array(w148, w143, w141, w137, w134) -> (w155:dbl[])
        n846 = Array To Cluster(array=w155) -> (cluster=→"Teperature Chart":T4)
        n847 = case shown="False" w132 {
          tunnel: w134 -> [w181 _]
          tunnel: [w181 w182] -> w133
          frame False {
            n848 = local write "Temperature 5"(w181) -> ()
          }
          frame True {
            n849 = local read "Temperature 5"() -> (w182:dbl)
          }
        }
        n850 = script code="MATLAB script"("T1"=w148, "T2"=w143, "T3"=w141, "T4"=w137, "T5"=w133) -> ()  [unwired: 1 in, 1 out]
      }
      n851 = while {
        stop <- w72 stop-if-true
        n852 = local read "Pump setpoint(ul/min) 1"() -> (w75:dbl)
        n853 = local read "Pump setpoint(ul/min) 2"() -> (w71:dbl)
        n854 = local read "Pump setpoint(ul/min) 3"() -> (w70:dbl)
        n855 = local read "Pump setpoint(ul/min) 4"() -> (w69:dbl)
        n856 = local read "Pump setpoint(ul/min) 5"() -> (w68:dbl)
        n857 = local read "Pump setpoint(ul/min) 6"() -> (w67:dbl)
        n858 = Build Array(w75, w71, w70, w69, w68, w67) -> (w76:dbl[])
        n859 = Array To Cluster(array=w76) -> (cluster=→"Pump Setpoints Chart":T4)
        n860 = Wait (ms)(milliseconds to wait=u32 5000) -> ()  [unwired: 1 out]
        n861 = local read "Stop"() -> (w72:bool)
      }
      n862 = while {
        tunnel: w52 -> [w64]
        stop <- w66 stop-if-true
        n863 = call-poly <vilib>:"Analog Read.vi"("Analog Channel"=u8 0, "LINX Resource"=w64) -> ("Voltage"=w63:dbl)  [unwired: 6 in, 3 out]
        "Phase_Sensor_voltage" <- w63
        n864 = Wait (ms)(milliseconds to wait=u32 300) -> ()  [unwired: 1 out]
        n865 = Build Array(w63) -> (w61:dbl[])
        n866 = Array To Cluster(array=w61) -> (cluster=→"Phase Sensor Chart":T4)
        n867 = local read "Stop"() -> (w66:bool)
      }
      n868 = while {
        tunnel: w52 -> [w125]
        stop <- w126 stop-if-true
        w81 = 270
        w92 = 600
        w101 = 600
        # "Read Pressure and Flowrate"
        n869 = local read "Stop"() -> (w126:bool)
        n870 = call-poly <vilib>:"Analog Read.vi"("AI Channel(s)"=i32[] [12, 13, 14, 15], "LINX Resource"=w125) -> ("Voltages"=w123:dbl[])  [unwired: 6 in, 3 out]
        n871 = Index Array(array=w123, index=3) -> (element=w115:dbl)
        n872 = Index Array(array=w123, index=2) -> (element=w116:dbl)
        n873 = Index Array(array=w123, index=1) -> (element=w117:dbl)
        n874 = Index Array(array=w123, index=0) -> (element=w118:dbl)
        n875 = call-poly <vilib>:"PID Control Input Filter.vi"("input"=w115) -> ("output"=w108:dbl)  [unwired: 4 in]
        n876 = call-poly <vilib>:"PID Control Input Filter.vi"("input"=w116) -> ("output"=w107:dbl)  [unwired: 4 in]
        n877 = call-poly <vilib>:"PID Control Input Filter.vi"("input"=w118) -> ("output"=w97:dbl)  [unwired: 4 in]
        n878 = call-poly <vilib>:"PID Control Input Filter.vi"("input"=w117) -> ("output"=w88:dbl)  [unwired: 4 in]
        n879 = Subtract(x=w97, y=0.065) -> (x-y=w98:dbl)
        n880 = Subtract(x=w88, y=0.065) -> (x-y=w89:dbl)
        n881 = Multiply(x=104.96 ("y"), y=w108) -> (x*y=w109:dbl)
        n882 = Multiply(x=104.96 ("y"), y=w107) -> (x*y=w112:dbl)
        n883 = Subtract(x=w109, y=24.077) -> (x-y=w79:dbl)
        n884 = Multiply(x=2, y=w101) -> (x*y=w103:i32)
        n885 = Divide(x=w103, y=3.3) -> (x/y=w99:dbl)
        n886 = Multiply(x=w98, y=w99) -> (x*y=w100:dbl)
        n887 = Subtract(x=w100, y=w101) -> (x-y=w83:dbl)
        n888 = Subtract(x=w112, y=24.077) -> (x-y=w80:dbl)
        n889 = Multiply(x=2, y=w92) -> (x*y=w94:i32)
        n890 = Divide(x=w94, y=3.3) -> (x/y=w90:dbl)
        n891 = Multiply(x=w89, y=w90) -> (x*y=w91:dbl)
        n892 = Subtract(x=w91, y=w92) -> (x-y=w82:dbl)
        n893 = Build Array(w83, w82) -> (w86:dbl[])
        n894 = Array To Cluster(array=w86) -> (cluster=→"Flowrate Chart":T4)
        n895 = Build Array(w80, w79) -> (w87:dbl[])
        n896 = local write "Flowrate Sensor 1"(w83) -> ()
        n897 = local write "Flowrate Sensor 2"(w82) -> ()
        n898 = local write "Pressure 1"(w80) -> ()
        n899 = local write "Pressure 2"(w79) -> ()
        n900 = Array To Cluster(array=w87) -> (cluster=→"Pressure Chart":T4)
        n901 = Wait (ms)(milliseconds to wait=u32 500) -> ()  [unwired: 1 out]
        n902 = script code="MATLAB script"("F1"=w83, "F2"=w82, "Pres1"=w80, "Pres2"=w79) -> ()  [unwired: 1 in, 1 out]
        n903 = Greater?(x=w79, y=w81) -> (0:w77:bool)
        n904 = Greater?(x=w80, y=w81) -> (0:w78:bool)
        n905 = case shown="False" w78 {
          frame False {
          }
          frame True {
            w130 = TRUE ("Stop")
            n906 = local write "System Error"(w130) -> ()
            n907 = local write "Stop"(w130) -> ()
            n908 = local write "Error Message"("Pressure Sensor 1 readings above 250psi") -> ()
            n909 = script code="system_error = 1;"() -> ()  [unwired: 1 in, 1 out]
          }
        }
        n910 = case shown="False" w77 {
          frame False {
          }
          frame True {
            w128 = TRUE ("Stop")
            n911 = local write "System Error"(w128) -> ()
            n912 = local write "Error Message"("Pressure Sensor 2 readings above 250psi") -> ()
            n913 = local write "Stop"(w128) -> ()
            n914 = script code="system_error = 1;"() -> ()  [unwired: 1 in, 1 out]
          }
        }
      }
    }
    frame #3 {
      # "Save and close xml and excel file"
      n915 = script code="if exist('xl_file','var') & exist('xlApp','var')\n  xlWorkbook.SaveAs(xl_file);\n  xlWorkbook.Close;\n  xlApp.Quit;\n  xlApp.delete;\nend"() -> ()  [unwired: 1 in, 1 out]
    }
    frame #4 {
      w1232 = string[] ["e", "f", "g", "h", "i", "j"]
      # "End communication to hardware"
      n916 = local read "Syringe_pump?"() -> (w1230:bool)
      n917 = local read "COMM Port:: Harvard Syringe Pump"() -> (w1231:refnum<visa-resource-name>)
      n918 = local read "IR Sensor Device"() -> (w1235:T2)
      n919 = call-poly <vilib>:"NI-845x Close Reference.vi"("device reference"=w1235) -> ()  [unwired: 10 in, 1 out]
      n920 = call <vilib>:"Close.vi"("LINX Resource"=w1236) -> ()  [unwired: 10 in, 1 out]
      n921 = local read "COMM Port :: Milligat Pumps"() -> (w1234:refnum<visa-resource-name>)
      n922 = Array Size(array=w1232) -> (size(s)=w1233:i32)
      n923 = case shown="True" w1230 {
        tunnel: w1231 -> [_ w1237]
        frame False {
        }
        frame True {
          n924 = call <instrlib>:"Stop Pump.vi"("VISA resource name"=w1237) -> ()  [unwired: 9 in, 2 out]
        }
      }
      n925 = for {
        N: w1233 -> [_]
        tunnel: w1232 -> [w1240] mode=indexing
        tunnel: w1234 -> [w1239]
        n926 = call "PumpStop.vi"("Pump Address"=w1240, "Pump COMM Port"=w1239) -> ()  [unwired: 9 in, 1 out]
        n927 = Wait (ms)(milliseconds to wait=u32 100) -> ()  [unwired: 1 out]
      }
    }
    frame #5 {
      # "Display Error Messages if necessary"
      n928 = local read "Error Message"() -> (w1241:string)
      n929 = One Button Dialog(message=w1241) -> ()  [unwired: 1 in, 1 out]
    }
  }
